vi "HEAT3.vi"() -> ()   [LabVIEW 2020]
uses:
  Control 2.ctl
  TDS_ProccesConfig.ctl
  rga_lv_85/SRSRGA85.llb/SRSRGAo RefNum.ctl
  <vilib>/Utility/miscctls.llb/LVRowAndColumnTypeDef.ctl
  <vilib>/Utility/sysdir.llb/System Directory Type.ctl
  <vilib>/Modbus/master/Create Master Instance (TCP).vi
  <vilib>/Utility/config.llb/Read Key (String).vi
  <vilib>/Waveform/WDTFileIO.llb/Export Waveforms To Spreadsheet File (1D).vi
  <vilib>/Utility/config.llb/Write Key (String).vi
  <vilib>/Modbus/master/Modbus Master.lvclass
  <vilib>/Utility/config.llb/NI_LVConfig.lvlib
panel:
  in  "TDS 2":T1={"Target Temp:"=10.0, "Target Ramp:"=1.0, "Ramp unit:"=1, "Temp. unit:"=0, "Target Ue [V]:"=500.0, "Target Ic [A]:"=2.0, "Heating Mode:"=FALSE, "PID Output:"=FALSE, "Regulation Type"=FALSE, "RGA Specifications"=[{"Mass"=2, "Noise Floor"=4, "CEM "=FALSE}], "Heating Recipe"=[]} {"RGA Specifications"."Noise Floor" min=0 max=7; "RGA Specifications"."Mass" min=1 max=300; "Temp. unit:" items=["K"=1, "C"=0]; "Ramp unit:" items=["/s", "/m", "/h"]}
  in  "TDS":T1={"Target Temp:"=10.0, "Target Ramp:"=1.0, "Ramp unit:"=1, "Temp. unit:"=0, "Target Ue [V]:"=500.0, "Target Ic [A]:"=2.0, "Heating Mode:"=FALSE, "PID Output:"=FALSE, "Regulation Type"=FALSE, "RGA Specifications"=[{"Mass"=2, "Noise Floor"=4, "CEM "=FALSE}], "Heating Recipe"=[]} {"RGA Specifications"."Noise Floor" min=0 max=7; "RGA Specifications"."Mass" min=1 max=300; "Temp. unit:" items=["K"=1, "C"=0]; "Ramp unit:" items=["/s", "/m", "/h"]}
  out "Remote:":bool
  out "heat_LastData":dbl[](array[numeric])
  out "size(s) 3":i32
  out "HEAT start time":timestamp=timestamp(3621395400.2120705 s since 1904-01-01)
  out "Array 2":waveform(dbl)[](array[waveform])
  out "Boolean":T2=TRUE
  out "stopped_loops":bool=TRUE
  in  "Tab Control":T3(tab)
  in  "Start 1":bool=TRUE
  in  "Clear ALL":bool
  out "Waveform Graph":waveform(dbl)[](graph)
  out "main Graph":T4(graph)={"heat_LastData[0]"=21.230000000000018, "heat_LastData[1]"=-273.15, "heat_LastData[2]"=0.0, "heat_LastData[3]"=0.0, "heat_LastData[4]"=0.0, "heat_LastData[5]"=0.0, "heat_LastData[6]"=0.0, "heat_LastData[7]"=0.0, "heat_LastData[8]"=0.0}
  in  "Clear ALL 2":bool
  in  "Start 2":bool=TRUE
  out "main Graph 2":T5(graph)
  in  "Tab Control 2":T6(tab)
  out "DualDC":bool
  out "Text Ring 5":u16(ring) items=["C/s", "C/m", "C/h"]
  out "Act. Ramp:":dbl=1.0
  in  "Save As Button":bool
  in  "Regulation TYpe":bool caption="Regulation Type:"
  in  "Target Ue [V]:":dbl=500.0
  in  "Target Ic [A]:":dbl=2.0
  in  "PID Output:":bool caption="PID Output Signal:"
  in  "Heating Mode:":bool
  out "Text Ring 3":u16(ring) items=["C/s", "C/m", "C/h"]
  out "Interlock:":bool
  out "Operate:":bool
  out "Text Ring":u16(ring) items=["K"=1, "C"=0]
  in  "OperateButton":bool caption="Operate:"
  out "Act. Temp:":dbl=24.100000000000023
  out "Act. P":dbl=100.0
  out "Act. I":dbl=50.0
  out "Act. D":dbl=1.0
  in  "Target Temp:":dbl=10.0
  in  "Target Ramp:":dbl=1.0
  in  "Temp. unit:":u16(ring) items=["K"=1, "C"=0]
  out "Act. Setpoint:":dbl=21.55000000000001
  out "Text Ring 2":u16(ring) items=["K"=1, "C"=0]
  in  "Ramp unit:":u16(ring)=1 items=["/s", "/m", "/h"]
  out "RES active:":bool
  out "EB active:":bool
  in  "Channel:":u16(ring)=7 items=["D1"=9, "D2"=11, "RTD"=13, "TC1"=5, "TC2"=7]
  in  "clean":bool
  out "Operate status::":bool[](array[boolean])=[FALSE, FALSE, FALSE, FALSE, FALSE, TRUE, TRUE, TRUE, FALSE, FALSE, FALSE, TRUE, FALSE, FALSE, FALSE, FALSE]
  in  "Shutter: CH1":bool caption="Shutter:"
  in  "ShutterControl":bool
  in  "Loadproject":bool
  in  "Saveproject":bool
  in  "Sampling time":dbl=250.0 format="%#_g ms"
  in  "Adv.RampControl":bool=TRUE
  out "Connected:":bool=TRUE
  in  "Reconect":bool
  out "Comunication error:":bool
  out "Text Ring 4":u16(ring) items=["C/s", "C/m", "C/h"]
  out "loop time":u32=499
  in  "Lock Button":bool
  in  "address":string="192.168.201.50"
  out "error out":errorcluster
  in  "Default Ramp:":dbl=60.0
  out "ResetActRamp":bool
  out "Uc Act.:":dbl
  out "Ic Act.:":dbl
  out "Uc Act.:":dbl
  out "Ic Act.:":dbl
  out "Ue Act.:":dbl
  out "Ie Act.:":dbl
  in  "Ie limit [mA]:":dbl
  in  "Ue limit [V]:":dbl
  in  "Ic limit [A]:":dbl
  in  "Uc limit [V]:":dbl
  in  "Ic limit:1":dbl caption="Ic limit [A]:"
  in  "Uc limit:1":dbl caption="Uc limit [V]:"
  out "new D":dbl=1.0
  out "new I":dbl=50.0
  out "new P":dbl=100.0
  in  "PID auto tab":string[][](table)
  in  "PID manual setting":string[][](table)=[["100", "50", "1"]]
  in  "Auto PID control":bool=TRUE
  out "New PID request":bool
  in  "Tab Control Duble Res":enum32{"HEAT3 Control", "HEAT3 Limits", "PID"}(tab)
  out "Text Ring 6":u16(ring) items=["K"=1, "C"=0]
  out "Act. Setpoint: 2":dbl=21.55000000000001 caption="Act. Setpoint:"
  in  "Target Ramp: 2":dbl=1.0 caption="Target Ramp:"
  in  "Target Temp: 2":dbl=10.0 caption="Target Temp:"
  out "Act. D 2":dbl=1.0 caption="Act. D"
  out "Act. I 2":dbl=50.0 caption="Act. I"
  out "Act. P 2":dbl=100.0 caption="Act. P"
  out "Act. Temp:":dbl=24.100000000000023
  out "Text Ring 7":u16(ring) items=["K"=1, "C"=0]
  out "Text Ring 8":u16(ring) items=["C/s", "C/m", "C/h"]
  in  "Target Ic [A]: 2":dbl=2.0 caption="Target Ic [A]:"
  out "Act. Ramp: 2":dbl=1.0 caption="Act. Ramp:"
  out "Text Ring 9":u16(ring) items=["C/s", "C/m", "C/h"]
  out "Text Ring 10":u16(ring) items=["K"=1, "C"=0]
  in  "OperateButton 2":bool caption="Operate:"
  in  "Regulation TYpe 2":bool caption="Regulation Type:"
  out "Operate: 2":bool caption="Operate:"
  out "Interlock: 2":bool caption="Interlock:"
  in  "Shutter: CH2":bool caption="Shutter:"
  in  "Uc limit:1 2":dbl caption="Uc limit [V]:"
  in  "Ic limit:1 2":dbl caption="Ic limit [A]:"
  out "Ic Act.: 2":dbl caption="Ic Act.:"
  out "Uc Act.: 2":dbl caption="Uc Act.:"
  out "New PID request 2":bool caption="New PID request"
  in  "Auto PID control 2":bool=TRUE caption="Auto PID control"
  in  "PID manual setting 2":string[][](table)=[["100", "50", "1"]] caption="PID manual setting"
  in  "PID auto tab 2":string[][](table) caption="PID auto tab"
  out "new P 2":dbl=100.0 caption="new P"
  out "new I 2":dbl=50.0 caption="new I"
  out "new D 2":dbl=1.0 caption="new D"
  in  "stop":bool=TRUE
  # "EB:"
  # "Process config.:"
  # "RES:"
  # "EB:"
  # "RES:"
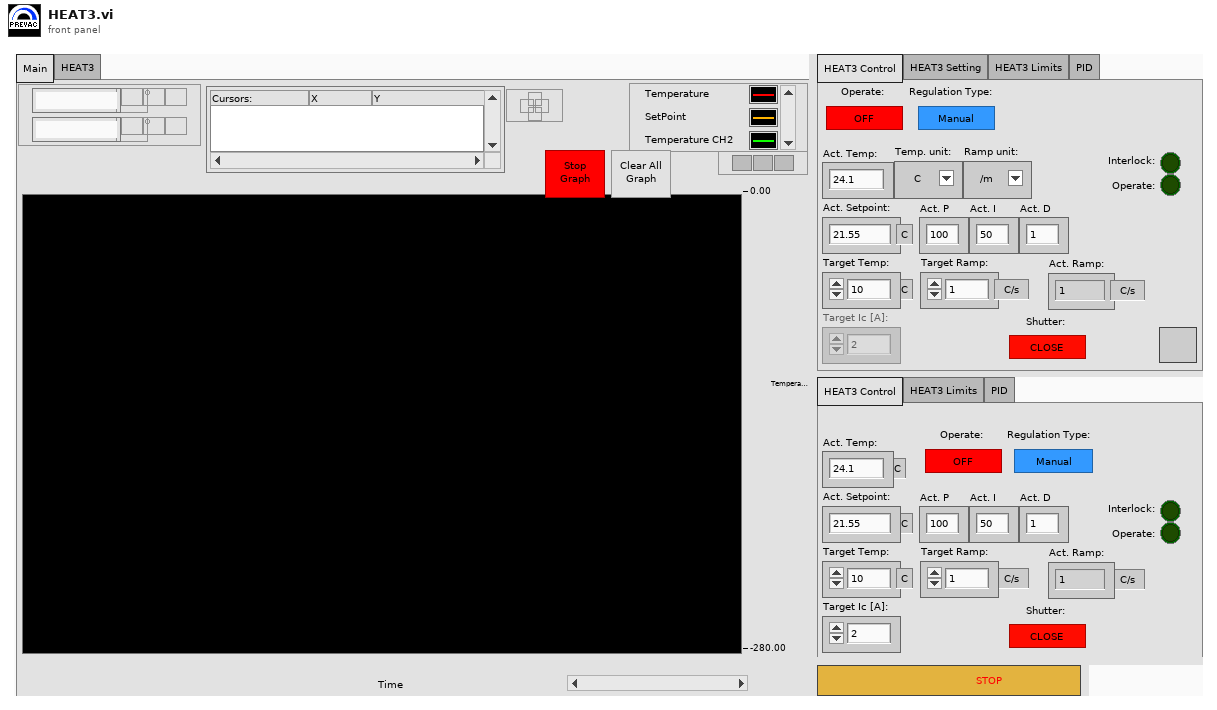
[diagram p1: front panel]
types:
  T1 = typedef "TDS_ProccesConfig.ctl" = cluster{"Target Temp:":dbl, "Target Ramp:":dbl, "Ramp unit:":u16, "Temp. unit:":u16, "Target Ue [V]:":dbl, "Target Ic [A]:":dbl, "Heating Mode:":bool, "PID Output:":bool, "Regulation Type":bool, "RGA Specifications":cluster{"Mass":i32, "Noise Floor":i32, "CEM ":bool}[], "Heating Recipe":cluster{"X":dbl, "Y":dbl}[]}
  T2 = typedef "Control 2.ctl" = bool
  T3 = enum32{"Main", "XY Graph", "Heating recepice", "RGA", "HEAT3"}
  T4 = cluster{"heat_LastData[0]":dbl, "heat_LastData[1]":dbl, "heat_LastData[2]":dbl, "heat_LastData[3]":dbl, "heat_LastData[4]":dbl, "heat_LastData[5]":dbl, "heat_LastData[6]":dbl, "heat_LastData[7]":dbl, "heat_LastData[8]":dbl}
  T5 = cluster{"[0]":dbl, "[1]":dbl, "[2]":dbl, "[3]":dbl}
  T6 = enum32{"HEAT3 Control", "HEAT3 Setting", "HEAT3 Limits", "PID"}
  T7 = typedef "SRSRGAo RefNum.ctl" = u16
  T8 = typedef "LVRowAndColumnTypeDef.ctl" = cluster{"Row":i32, "Column":i32}
  T9 = enum8{"Enabled", "Disabled", "Disabled and Grayed Out"}
  T10 = cluster{"Name":string, "Color":u32, "Style":u8, "Point Style":u8, "Name Visible":bool, "Allow Drag":bool, "Cursor Mode":u32, "Plot":i32, "Index":i32, "Position":cluster{"X":dbl, "Y":dbl}, "X Scale":u32, "Y Scale":u32, "Watch Plots":i32[], "Watch All Plots":bool, "Plot Area":i32, "Label Offset":cluster{"X":dbl, "Y":dbl}}
  T11 = cluster{"heat_LastData[0]":dbl, "heat_LastData[1]":dbl, "heat_LastData[2]":dbl, "heat_LastData[3]":dbl, "heat_LastData[4]":dbl, "heat_LastData[5]":dbl, "heat_LastData[6]":dbl, "heat_LastData[7]":dbl, "heat_LastData[8]":dbl}[]
  T12 = enum16{"open", "replace", "create", "open or create", "replace or create", "replace or create with confirmation"}
  T13 = cluster{"[0]":dbl, "[1]":dbl, "[2]":dbl, "[3]":dbl}[]
  T14 = typedef "LVRectTypeDef.ctl" = cluster{"Left":i16, "Top":i16, "Right":i16, "Bottom":i16}
  T15 = typedef "NI_LVConfig.lvlib/Config Data RefNum.ctl" = refnum<k1>
  T16 = typedef "System Directory Type.ctl" = i32
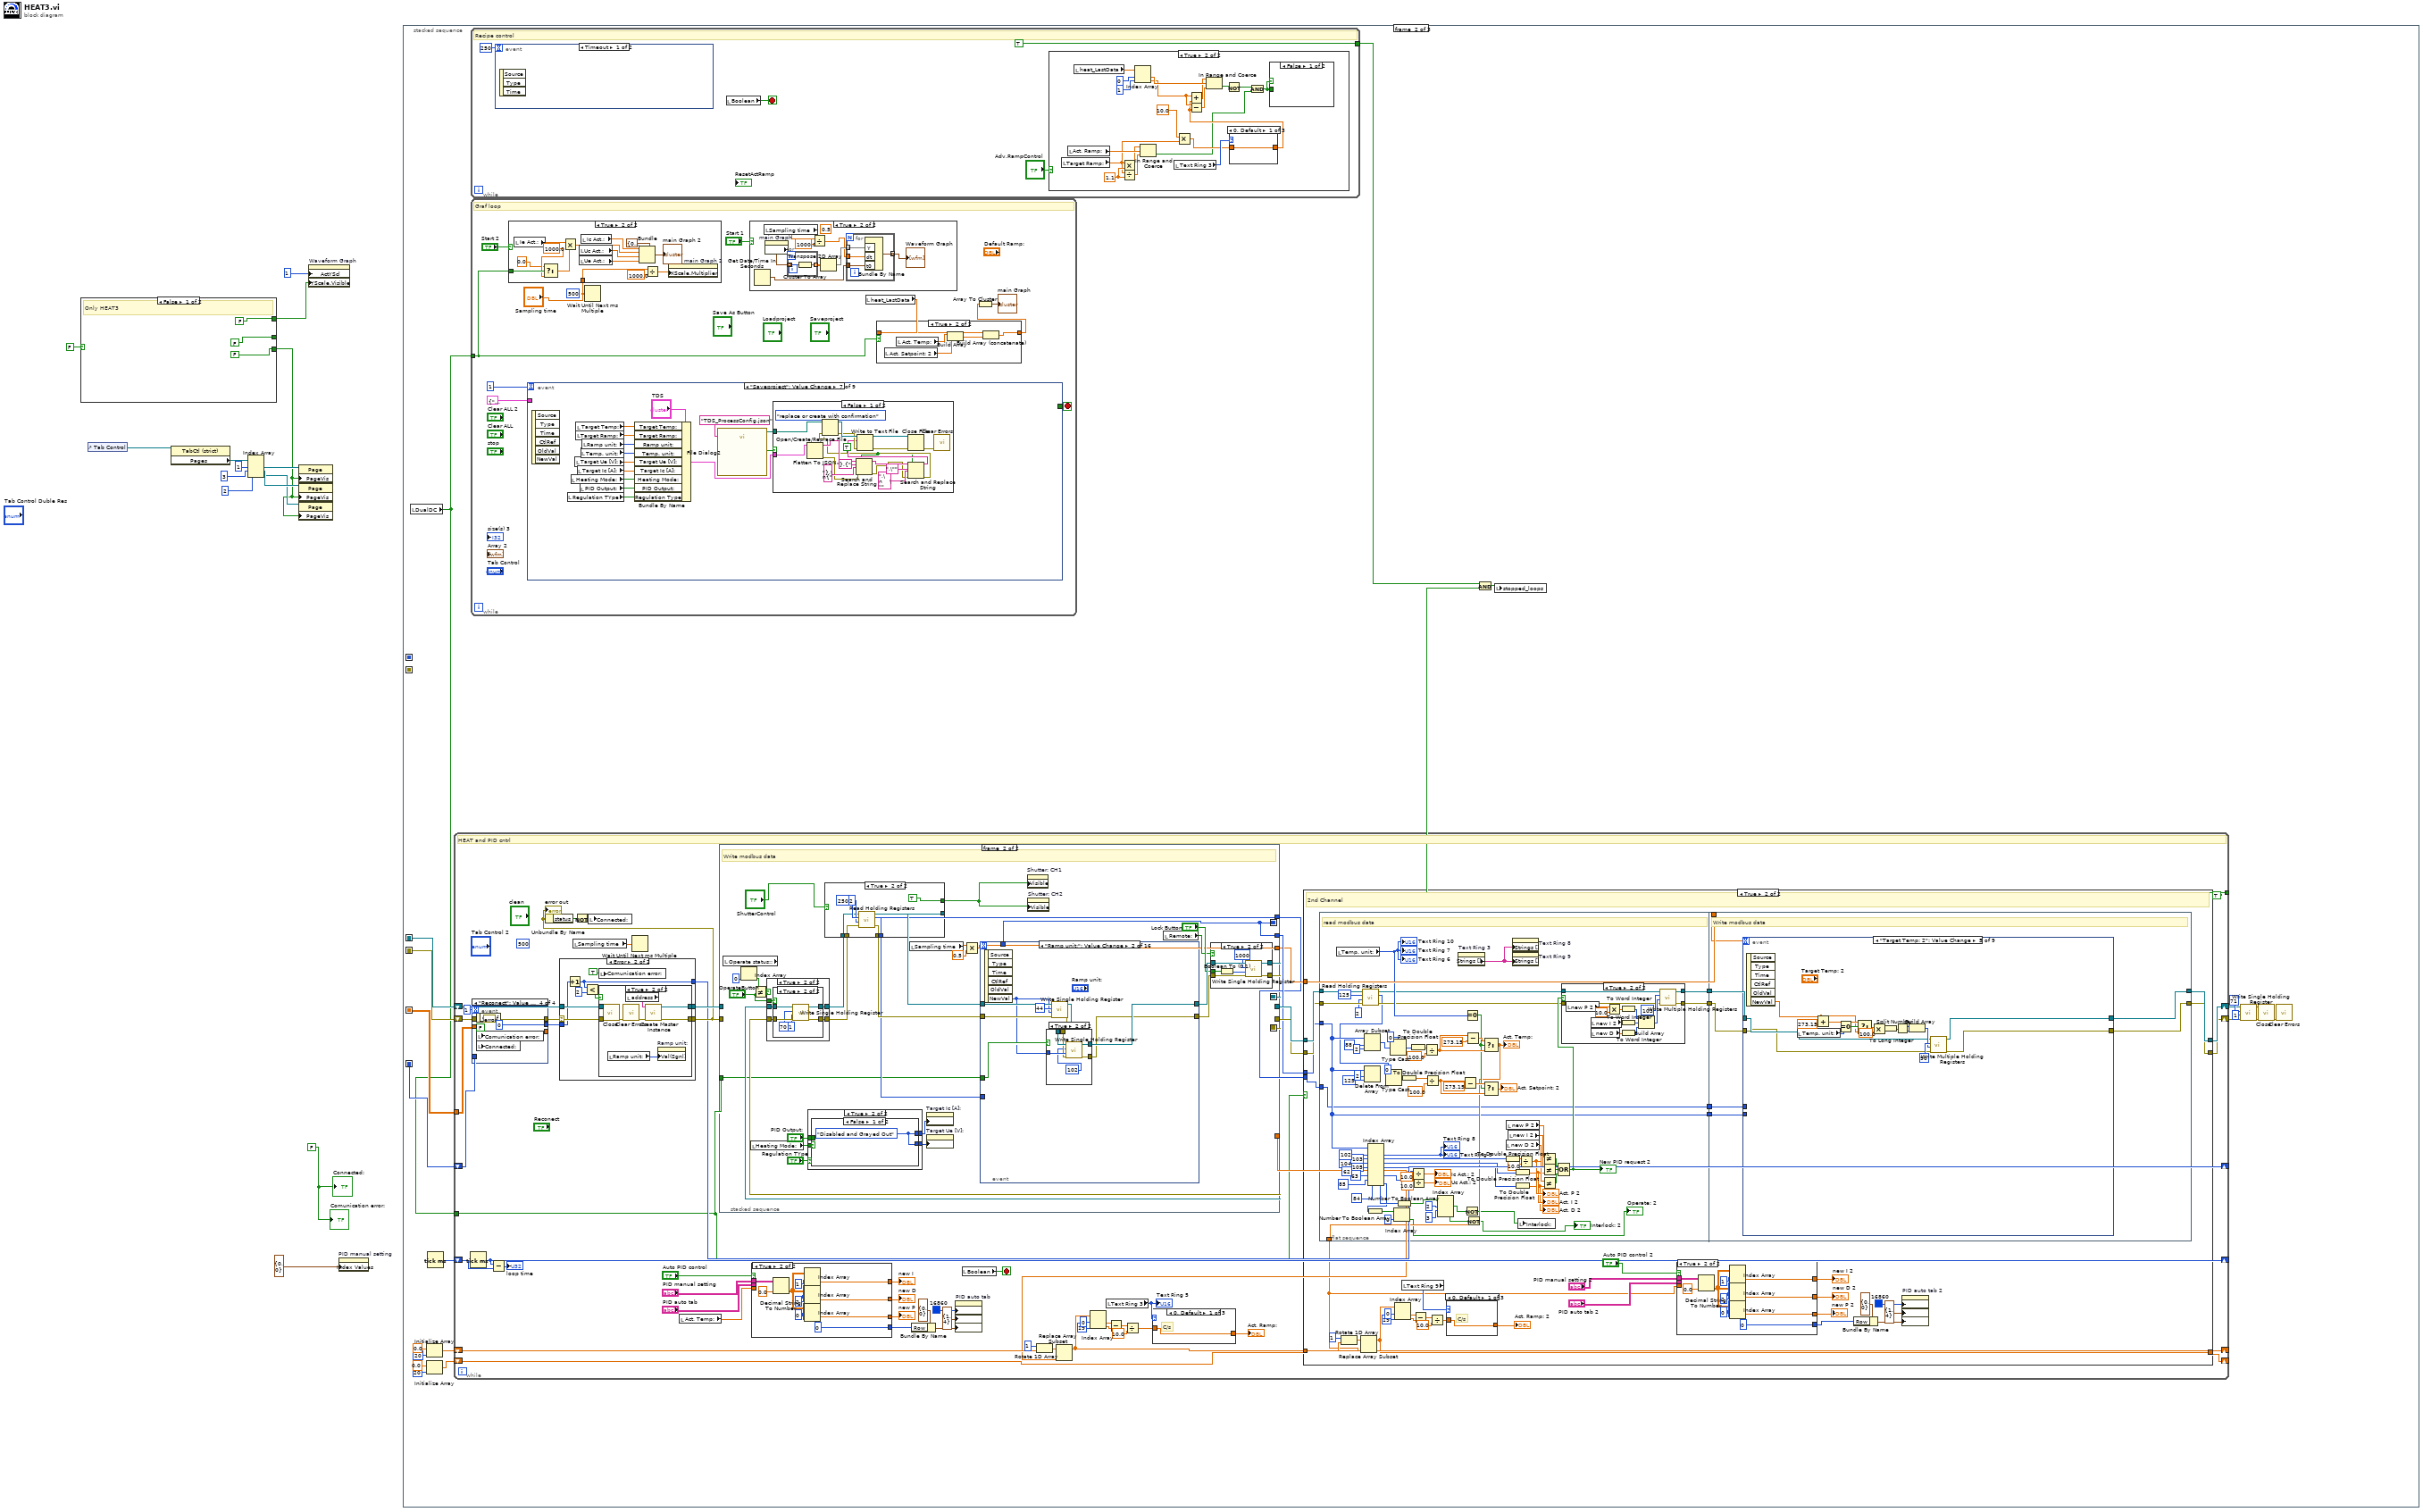
[diagram p0: block diagram]
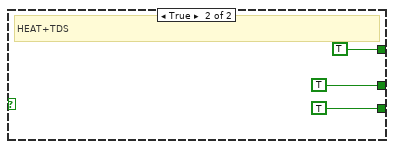
[diagram p2: hidden frame]
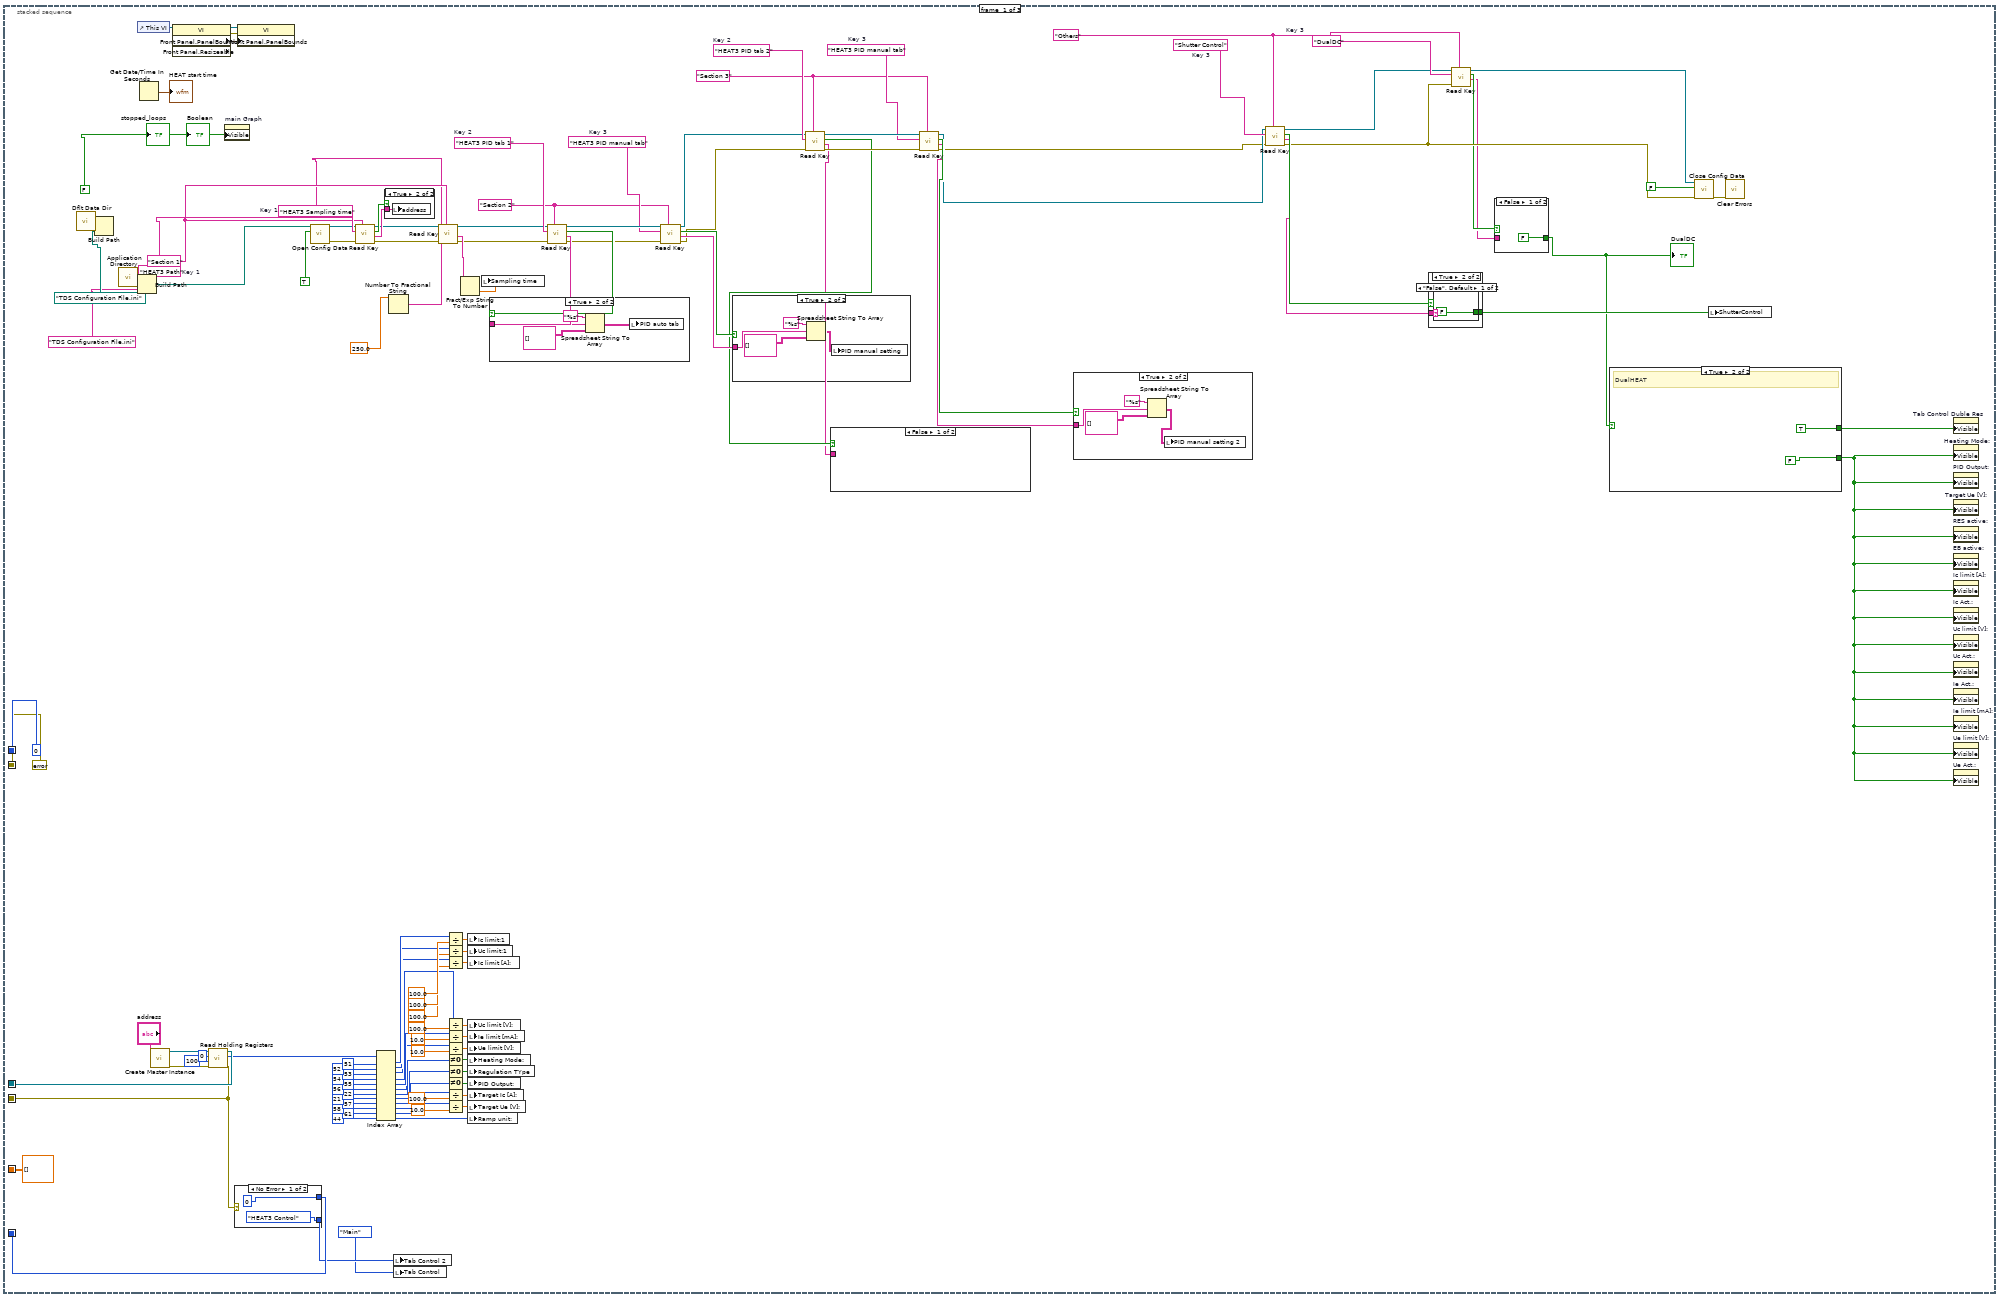
[diagram p3: hidden frame]
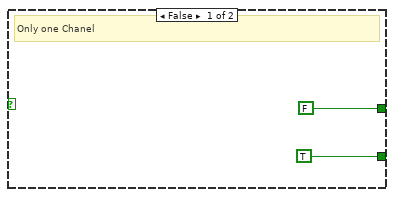
[diagram p4: hidden frame]
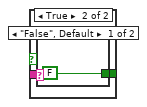
[diagram p5: hidden frame]
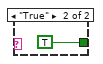
[diagram p6: hidden frame]
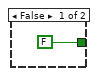
[diagram p7: hidden frame]
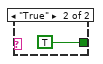
[diagram p8: hidden frame]
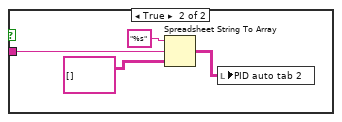
[diagram p10: hidden frame]
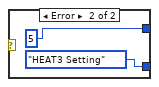
[diagram p13: hidden frame]
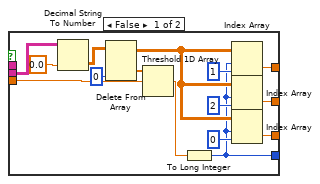
[diagram p16: hidden frame]
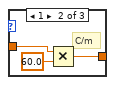
[diagram p17: hidden frame]
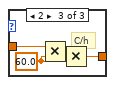
[diagram p18: hidden frame]
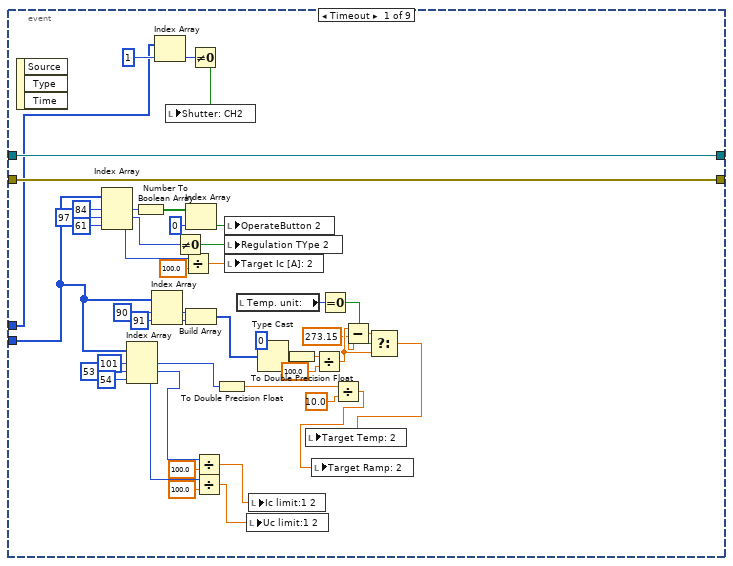
[diagram p20: hidden frame]
diagram:
  w14 = FALSE ("Connected:")
  n1 = case shown="False" FALSE {
    tunnel: [FALSE ("Visible") TRUE ("Visible")] -> _
    tunnel: [FALSE ("Page Visible") TRUE ("Page Visible")] -> w1
    tunnel: [FALSE ("Visible") TRUE ("Visible")] -> w4
    frame False {
      # "Only HEAT3"
    }
    frame True {
      # "HEAT+TDS"
    }
  }
  n2 = control-ref of="Tab Control"() -> (w8:refnum<vi>)
  n3 = property class="TabCtl (strict)"(reference=w8) -> ("Pages"=w11:refnum<vi>[])  [unwired: 1 in, 2 out]
  n4 = Index Array(array=w11, index #1=1 ("index"), index #2=3 ("index"), index #3=2 ("index")) -> (element #1=w9:refnum<vi>, element #2=w6:refnum<vi>, element #3=w2:refnum<vi>)
  n5 = property class="Page"(reference=w9, "PageVis"=w1) -> ()  [unwired: 1 in, 2 out]
  n6 = property class="Page"(reference=w6, "PageVis"=w1) -> ()  [unwired: 1 in, 2 out]
  n7 = property class="Page"(reference=w2, "PageVis"=w1) -> ()  [unwired: 1 in, 2 out]
  n8 = property on="Waveform Graph" class="WFGraph (strict)"("ActYScl"=1, "YScale.Visible"=w4) -> ()  [unwired: 2 in, 2 out]
  n9 = property on="PID manual setting" class="Tbl (strict)"("Index Values"=cluster{"Row":u32, "Column":u32} {"Row"=0, "Column"=0}) -> ()  [unwired: 2 in, 2 out]
  n10 = stacked-sequence {
    seq-local: [w123 _ _] -> [_ w198 _]
    seq-local: [w76 _ _] -> [_ w197 _]
    seq-local: [dbl[][] [] _ _] -> [_ w184 _]
    seq-local: [T7 0 ("SRSRGA Refnum") _ _] -> [_ _ _]
    seq-local: [errorcluster {"status"=FALSE, "code"=0, "source"=""} ("error out") _ _] -> [_ _ _]
    seq-local: [w75 _ _] -> [_ w189 _]
    frame #0 {
      w29 = "DualDC"  # Key 3
      w30 = "Others" ("section")
      w37 = "Shutter Control"  # Key 3
      w44 = "HEAT3 PID manual tab"  # Key 3
      w47 = "HEAT3 PID tab 2"  # Key 2
      w34 = "Section 3" ("section")
      w53 = "HEAT3 Sampling time"  # Key 1
      w68 = "HEAT3 PID manual tab"  # Key 3
      w74 = "HEAT3 PID tab 1"  # Key 2
      w65 = "Section 2" ("section")
      w130 = "HEAT3 Path"  # Key 1
      w54 = "Section 1" ("section")
      w63 = FALSE ("Boolean")
      n11 = call <vilib>:"Dflt Data Dir.vi"() -> ("App:Default Data Directory"=w135:path)
      n12 = Build Path(base path=w135, name or relative path=path "TDS Configuration File.ini" ("default name")) -> ()  [unwired: 1 out]
      n13 = call <vilib>:"Application Directory.vi"() -> ("Application Directory"=w60:path)
      n14 = control-ref of="This VI"() -> (w140:refnum<vi>)
      n15 = Build Path(base path=w60, name or relative path="TDS Configuration File.ini") -> (appended path=w59:path)
      n16 = Get Date/Time In Seconds() -> (seconds since 1Jan1904=→"HEAT start time":timestamp)
      n17 = call-poly <vilib>:"Create Master Instance.vi"("address"="address") -> ("error out"=w124:errorcluster, "TCP master instance"=w125:refnum<class "Modbus Master.lvclass">)  [unwired: 9 in]
      n18 = property class="VI" props=["Front Panel.PanelBounds", "Front Panel.Resizeable"](reference=w140) -> (reference out=w138:refnum<vi>, error out=w137:errorcluster, "Front Panel.PanelBounds"=w139:T14)  [unwired: 1 in, 1 out]
      n19 = call-dynamic "Read Holding Registers.vi"("error in (no error)"=w124, "number of holding registers"=u16 100, "starting address"=u16 0, "Modbus master in"=w125) -> ("error out"=w76:errorcluster, "register values"=w118:u16[], "Modbus master out"=w123:refnum<class "Modbus Master.lvclass">)  [unwired: 5 in]
      n20 = property on="main Graph" class="WFChart (strict)"("Visible"=w63) -> ()  [unwired: 2 in, 2 out]
      n21 = case shown="No Error" w76 {
        tunnel: [0 5] -> w75
        tunnel: [T6."HEAT3 Control" ("Tab Control 2") T6."HEAT3 Setting" ("Tab Control 2")] -> w71
        frame No Error {
        }
        frame Error {
        }
      }
      n22 = property class="VI"(reference=w138, error in=w137, "Front Panel.PanelBounds"=w139) -> ()  [unwired: 2 out]
      n23 = call <vilib>:"Open Config Data.vi"("create file if necessary (T)"=TRUE ("create file if necessary? (T)"), "configuration file path"=w59) -> ("error out"=w128:errorcluster, "refnum"=w129:T15)  [unwired: 7 in, 1 out]
      n24 = call-poly <vilib>:"Read Key.vi"("section"=w54, "error in (no error)"=w128, "key"=w130, "refnum"=w129) -> ("error out"=w50:errorcluster, "value"=w132:string, "found?"=w131:bool, "refnum out"=w52:T15)  [unwired: 2 in, 2 out]
      n25 = Index Array(array=w118, index #1=51 ("index"), index #2=52 ("index"), index #3=53 ("index"), index #4=54 ("index"), index #5=55 ("index"), index #6=56 ("index"), index #7=22 ("index"), index #8=21 ("index"), index #9=57 ("index"), index #10=58 ("index"), index #11=61 ("index"), index #12=44 ("index")) -> (element #1=w109:u16, element #2=w108:u16, element #3=w107:u16, element #4=w95:u16, element #5=w106:u16, element #6=w94:u16, element #7=w98:u16, element #8=w48:u16, element #9=w87:u16, element #10=w80:u16, element #11=w79:u16, element #12=w77:u16)
      n26 = case shown="True" w131 {
        tunnel: w132 -> [_ w177]
        frame False {
        }
        frame True {
          n27 = local write "address"(w177) -> ()
        }
      }
      n28 = Number To Fractional String(number=250.0) -> (F-format string=w57:string)  [unwired: 3 in]
      n29 = local write "Tab Control 2"(w71) -> ()
      n30 = local write "Tab Control"(T3."Main" ("Tab Control")) -> ()
      n31 = call-poly <vilib>:"Read Key.vi"("section"=w54, "error in (no error)"=w50, "default value"=w57, "key"=w53, "refnum"=w52) -> ("error out"=w49:errorcluster, "value"=w56:string, "refnum out"=w51:T15)  [unwired: 1 in, 3 out]
      n32 = Divide(x=w109, y=100.0) -> (x/y=w105:dbl)
      n33 = Divide(x=w108, y=100.0) -> (x/y=w104:dbl)
      n34 = Divide(x=w107, y=100.0) -> (x/y=w103:dbl)
      n35 = Divide(x=w95, y=100.0) -> (x/y=w102:dbl)
      n36 = Divide(x=w106, y=10.0) -> (x/y=w101:dbl)
      n37 = Divide(x=w94, y=10.0) -> (x/y=w100:dbl)
      n38 = Not Equal To 0?(x=w98) -> (x != 0?=w97:bool)
      n39 = Not Equal To 0?(x=w48) -> (x != 0?=w91:bool)
      n40 = Not Equal To 0?(x=w87) -> (x != 0?=w90:bool)
      n41 = Divide(x=w80, y=100.0) -> (x/y=w84:dbl)
      n42 = Divide(x=w79, y=10.0) -> (x/y=w83:dbl)
      n43 = Fract/Exp String To Number(string=w56) -> (number=w55:dbl)  [unwired: 3 in, 1 out]
      n44 = local write "Ic limit:1"(w105) -> ()
      n45 = local write "Uc limit:1"(w104) -> ()
      n46 = local write "Ic limit [A]:"(w103) -> ()
      n47 = local write "Uc limit [V]:"(w102) -> ()
      n48 = local write "Ie limit [mA]:"(w101) -> ()
      n49 = local write "Ue limit [V]:"(w100) -> ()
      n50 = local write "Heating Mode:"(w97) -> ()
      n51 = local write "Regulation TYpe"(w91) -> ()
      n52 = local write "PID Output:"(w90) -> ()
      n53 = local write "Target Ic [A]:"(w84) -> ()
      n54 = local write "Target Ue [V]:"(w83) -> ()
      n55 = local write "Ramp unit:"(w77) -> ()
      n56 = local write "Sampling time"(w55) -> ()
      n57 = call-poly <vilib>:"Read Key.vi"("section"=w65, "error in (no error)"=w49, "key"=w74, "refnum"=w51) -> ("error out"=w69:errorcluster, "value"=w72:string, "found?"=w73:bool, "refnum out"=w70:T15)  [unwired: 2 in, 2 out]
      n58 = case shown="True" w73 {
        tunnel: w72 -> [_ w172]
        frame False {
        }
        frame True {
          n59 = Spreadsheet String To Array(format string="%s", spreadsheet string=w172, array type (2D Dbl)=string[][] [] ("PID auto tab")) -> (array=w169:string[][])  [unwired: 1 in]
          n60 = local write "PID auto tab"(w169) -> ()
        }
      }
      n61 = call-poly <vilib>:"Read Key.vi"("section"=w65, "error in (no error)"=w69, "key"=w68, "refnum"=w70) -> ("error out"=w42:errorcluster, "value"=w66:string, "found?"=w67:bool, "refnum out"=w43:T15)  [unwired: 2 in, 2 out]
      n62 = case shown="True" w67 {
        tunnel: w66 -> [_ w166]
        frame False {
        }
        frame True {
          n63 = Spreadsheet String To Array(format string="%s", spreadsheet string=w166, array type (2D Dbl)=string[][] [] ("PID auto tab")) -> (array=w165:string[][])  [unwired: 1 in]
          n64 = local write "PID manual setting"(w165) -> ()
        }
      }
      n65 = call-poly <vilib>:"Read Key.vi"("section"=w34, "error in (no error)"=w42, "key"=w47, "refnum"=w43) -> ("error out"=w45:errorcluster, "value"=w40:string, "found?"=w41:bool, "refnum out"=w46:T15)  [unwired: 2 in, 2 out]
      n66 = case shown="False" w41 {
        tunnel: w40 -> [_ w164]
        frame False {
        }
        frame True {
          n67 = Spreadsheet String To Array(format string="%s", spreadsheet string=w164, array type (2D Dbl)=string[][] [] ("PID auto tab")) -> (array=w161:string[][])  [unwired: 1 in]
          n68 = local write "PID auto tab 2"(w161) -> ()
        }
      }
      n69 = call-poly <vilib>:"Read Key.vi"("section"=w34, "error in (no error)"=w45, "key"=w44, "refnum"=w46) -> ("error out"=w35:errorcluster, "value"=w38:string, "found?"=w39:bool, "refnum out"=w36:T15)  [unwired: 2 in, 2 out]
      n70 = case shown="True" w39 {
        tunnel: w38 -> [_ w158]
        frame False {
        }
        frame True {
          n71 = Spreadsheet String To Array(format string="%s", spreadsheet string=w158, array type (2D Dbl)=string[][] [] ("PID auto tab")) -> (array=w157:string[][])  [unwired: 1 in]
          n72 = local write "PID manual setting 2"(w157) -> ()
        }
      }
      n73 = call-poly <vilib>:"Read Key.vi"("section"=w30, "error in (no error)"=w35, "key"=w37, "refnum"=w36) -> ("error out"=w26:errorcluster, "value"=w32:string, "found?"=w33:bool, "refnum out"=w28:T15)  [unwired: 2 in, 2 out]
      n74 = case shown="True" w33 {
        tunnel: w32 -> [_ w154]
        tunnel: [FALSE ("Page Visible") w153] -> w31
        frame False {
        }
        frame True {
          n75 = case shown="\"False\", Default" w154 {
            tunnel: [FALSE ("Page Visible") TRUE ("Page Visible")] -> w153
            frame "False", Default {
            }
            frame "True" {
            }
          }
        }
      }
      n76 = call-poly <vilib>:"Read Key.vi"("section"=w30, "error in (no error)"=w26, "key"=w29, "refnum"=w28) -> ("value"=w24:string, "found?"=w25:bool, "refnum out"=w27:T15)  [unwired: 2 in, 3 out]
      n77 = case shown="False" w25 {
        tunnel: w24 -> [_ w149]
        tunnel: [FALSE ("Page Visible") w148] -> w21
        frame False {
        }
        frame True {
          n78 = case shown="\"False\", Default" w149 {
            tunnel: [FALSE ("Page Visible") TRUE ("Page Visible")] -> w148
            frame "False", Default {
            }
            frame "True" {
            }
          }
        }
      }
      "DualDC" <- w21
      n79 = case shown="True" w21 {
        tunnel: [FALSE ("Page Visible") TRUE ("Page Visible")] -> w23
        tunnel: [TRUE ("Page Visible") FALSE ("Page Visible")] -> w22
        frame False {
          # "Only one Chanel"
        }
        frame True {
          # "DualHEAT"
        }
      }
      n80 = call <vilib>:"Close Config Data.vi"("error in (no error)"=w26, "write file if changed (T)"=FALSE ("write configuration file? (T)"), "refnum"=w27) -> ("error out"=w62:errorcluster)  [unwired: 8 out]
      n81 = local write "ShutterControl"(w31) -> ()
      n82 = call <vilib>:"Clear Errors.vi"("error in (no error)"=w62) -> ()  [unwired: 5 in, 2 out]
      n83 = property on="Tab Control Duble Res" class="TabCtl (strict)"("Visible"=w23) -> ()  [unwired: 2 in, 2 out]
      n84 = property on="Heating Mode:" class="Bool (strict)"("Visible"=w22) -> ()  [unwired: 2 in, 2 out]
      n85 = property on="PID Output:" class="Bool (strict)"("Visible"=w22) -> ()  [unwired: 2 in, 2 out]
      n86 = property on="Target Ue [V]:" class="DigNum (strict)"("Visible"=w22) -> ()  [unwired: 2 in, 2 out]
      n87 = property on="RES active:" class="Bool (strict)"("Visible"=w22) -> ()  [unwired: 2 in, 2 out]
      n88 = property on="EB active:" class="Bool (strict)"("Visible"=w22) -> ()  [unwired: 2 in, 2 out]
      n89 = property on="Ic limit [A]:" class="DigNum (strict)"("Visible"=w22) -> ()  [unwired: 2 in, 2 out]
      n90 = property on="Ic Act.:" class="DigNum (strict)"("Visible"=w22) -> ()  [unwired: 2 in, 2 out]
      n91 = property on="Uc limit [V]:" class="DigNum (strict)"("Visible"=w22) -> ()  [unwired: 2 in, 2 out]
      n92 = property on="Uc Act.:" class="DigNum (strict)"("Visible"=w22) -> ()  [unwired: 2 in, 2 out]
      n93 = property on="Ie Act.:" class="DigNum (strict)"("Visible"=w22) -> ()  [unwired: 2 in, 2 out]
      n94 = property on="Ie limit [mA]:" class="DigNum (strict)"("Visible"=w22) -> ()  [unwired: 2 in, 2 out]
      n95 = property on="Ue limit [V]:" class="DigNum (strict)"("Visible"=w22) -> ()  [unwired: 2 in, 2 out]
      n96 = property on="Ue Act.:" class="DigNum (strict)"("Visible"=w22) -> ()  [unwired: 2 in, 2 out]
      "stopped_loops" <- w63
      "Boolean" <- w63
    }
    frame #1 {
      n97 = local read "DualDC"() -> (w178:bool)
      n98 = Initialize Array(0.0 ("element"), 20 ("dimension size")) -> (w179:dbl[])
      n99 = Initialize Array(0.0 ("element"), 20 ("dimension size")) -> (w186:dbl[])
      n100 = Tick Count (ms)() -> (millisecond timer value=w185:u32)
      n101 = while {
        tunnel: [TRUE] -> w182
        shift-right: [w206] -> w193
        shift-left: w197 -> [w232]
        shift-right: [w208] -> w194
        shift-left: w198 -> [w240]
        shift-right: [w236] -> _
        shift-left: w185 -> [w235]
        shift-right: [w225] -> _
        shift-left: w189 -> [w230]
        tunnel: w184 -> [w237]
        shift-right: [w221] -> _
        shift-left: w186 -> [w224]
        tunnel: w178 -> [w204]
        shift-right: [w202] -> _
        shift-left: w179 -> [w203]
        stop <- w253 stop-if-true
        (unwired) u32 500 ("millisecond multiple")
        # "HEAT and PID cntrl"
        n102 = Tick Count (ms)() -> (millisecond timer value=w236:u32)
        n103 = event shown="[3] \"Reconect\": Value Change" {
          selector: _ -> [_ _ _ _]
          dyn-events: _ -> [_ _ _ _]
          timeout: 1 -> [_ _ _ _]
          tunnel: w237 -> [w971 _ _ _]
          tunnel: [w969 dbl[][] [] _ _] -> _
          tunnel: [w968 w974 errorcluster {"status"=TRUE, "code"=0, "source"="Connect to\nnew IP addres"} ("error constant") errorcluster {"status"=TRUE, "code"=0, "source"="Rconnecting"} ("error constant")] -> w231
          tunnel: w232 -> [w968 w974 _ _]
          tunnel: [w967 w973 0 0] -> w229
          tunnel: w230 -> [w967 w973 _ _]
          event Timeout {
            n104 = event-data() -> ()  [unwired: 1 in, 1 out]
            n105 = Select(t=w971, s=FALSE ("build array of data?"), f=dbl[][] []) -> (s? t:f=w969:dbl[][])
          }
          event "clean": Value Change {
            n106 = event-data() -> ()  [unwired: 1 in, 1 out]
            n107 = Get Date/Time In Seconds() -> (seconds since 1Jan1904=w975:timestamp)
            n108 = local write "HEAT start time"(w975) -> ()
            n109 = local write "clean"(FALSE ("clc graph")) -> ()
          }
          event "address": Value Change {
            n110 = event-data() -> ()  [unwired: 1 in, 1 out]
          }
          event "Reconect": Value Change {
            w980 = FALSE ("Connected:")
            n111 = event-data() -> ()  [unwired: 1 in, 1 out]
            n112 = local write "Comunication error:"(w980) -> ()
            n113 = local write "Connected:"(w980) -> ()
          }
        }
        n114 = Subtract(x=w236, y=w235) -> (x-y=→"loop time":u32)
        n115 = case shown="Error" w231 {
          selector: w231 -> [w987 w996]
          tunnel: [w987 w993] -> w227
          tunnel: w240 -> [w986 w995]
          tunnel: [w986 w994] -> w239
          tunnel: w229 -> [_ w991]
          tunnel: [0 w990] -> w225
          frame No Error {
            w983 = FALSE
            n116 = Not(x=w983) -> (.not. x?=w984:bool)
            n117 = local write "Comunication error:"(w983) -> ()
            n118 = local write "Connected:"(w984) -> ()
          }
          frame Error {
            n119 = Increment(x=w991) -> (x+1=w990:i32)
            n120 = Less?(x=w990, y=2) -> (x < y?=w989:bool)
            n121 = local write "Comunication error:"(TRUE) -> ()
            n122 = case shown="True" w989 {
              tunnel: w996 -> [w997 w1006]
              tunnel: w995 -> [w998 w1005]
              tunnel: [w998 w1003] -> w994
              tunnel: [w997 w1002] -> w993
              frame False {
              }
              frame True {
                n123 = call-dynamic "Close.vi"("error in (no error)"=w1006, "Modbus master in"=w1005) -> ("error out"=w1001:errorcluster)  [unwired: 9 in]
                n124 = local read "Ramp unit:"() -> (w999:u16)
                n125 = call <vilib>:"Clear Errors.vi"("error in (no error)"=w1001) -> ("error out"=w1000:errorcluster)  [unwired: 5 in, 1 out]
                n126 = local read "address"() -> (w1004:string)
                n127 = call-poly <vilib>:"Create Master Instance.vi"("error in (no error)"=w1000, "address"=w1004) -> ("error out"=w1002:errorcluster, "TCP master instance"=w1003:refnum<class "Modbus Master.lvclass">)  [unwired: 8 in]
                n128 = property on="Ramp unit:" class="Ring (strict)"("Val(Sgnl)"=w999) -> ()  [unwired: 2 in, 2 out]
              }
            }
          }
        }
        "error out" <- w227
        n129 = Unbundle By Name(w227) -> ("status"=w228:bool)
        n130 = local read "Sampling time"() -> (w211:dbl)
        n131 = Not(x=w228) -> (.not. x?=w226:bool)
        n132 = local write "Connected:"(w226) -> ()
        n133 = Wait Until Next ms Multiple(millisecond multiple=w211) -> ()  [unwired: 1 out]
        n134 = local read "Act. Temp:"() -> (w241:dbl)
        n135 = stacked-sequence {
          seq-local: [w589 _] -> [_ w677]
          seq-local: [w588 _] -> [_ w676]
          seq-local: [w573 _] -> [_ w662]
          tunnel: w239 -> [w587 _]
          tunnel: w227 -> [w586 _]
          tunnel: [_ w669] -> w209
          tunnel: [_ w667] -> w207
          tunnel: [w577 _] -> w210
          tunnel: [_ w662] -> w205
          tunnel: w204 -> [w572 w653]
          tunnel: [_ w661] -> w201
          tunnel: [_ w656] -> w200
          frame #0 {
            # "read modbus data"
            n136 = call-dynamic "Read Holding Registers.vi"("error in (no error)"=w586, "number of holding registers"=u16 1, "starting address"=u16 1151, "Modbus master in"=w587) -> ("error out"=w584:errorcluster, "register values"=w578:u16[], "Modbus master out"=w585:refnum<class "Modbus Master.lvclass">)  [unwired: 5 in]
            n137 = Index Array(array=w578) -> (element=w579:u16)  [unwired: 1 in]
            n138 = Not Equal To 0?(x=w579) -> (x != 0?=w580:bool)
            "Remote:" <- w580
            n139 = case shown="False" w580 {
              tunnel: [T9."Disabled and Grayed Out" ("Disabled") T9."Enabled" ("Disabled")] -> w581
              frame False {
                n140 = local write "Lock Button"(FALSE ("Lock Button")) -> ()
              }
              frame True {
              }
            }
            n141 = local read "Act. Setpoint:"() -> (w605:dbl)
            n142 = disable-structure shown="Disabled" {
              disable-tunnel: [w634 u16 2] -> w610
              frame Disabled {
                n143 = Decrement(x="Channel:") -> (x-1=w634:u16)
              }
              frame Enabled {
              }
            }
            n144 = local read "Act. Temp:"() -> (w577:dbl)
            n145 = call-dynamic "Read Holding Registers.vi"("error in (no error)"=w584, "number of holding registers"=u16 1, "starting address"=u16 0, "Modbus master in"=w585) -> ("error out"=w622:errorcluster, "register values"=w594:u16[], "Modbus master out"=w623:refnum<class "Modbus Master.lvclass">)  [unwired: 5 in]
            n146 = property on="Lock Button" class="Bool (strict)"("DisabledEnum"=w581) -> ()  [unwired: 2 in, 2 out]
            n147 = call-dynamic "Read Holding Registers.vi"("error in (no error)"=w622, "number of holding registers"=u16 2, "starting address"=w610, "Modbus master in"=w623) -> ("error out"=w628:errorcluster, "register values"=w608:u16[], "Modbus master out"=w629:refnum<class "Modbus Master.lvclass">)  [unwired: 5 in]
            n148 = call "Modbus_Get_Status_list.vi"("register values"=w594) -> ("Boolean"=w602:bool, "Boolean 2"=→"Operate:":bool, "Boolean array"=→"Operate status::":bool[])  [unwired: 8 in]
            n149 = Build Array(w577, w605) -> (→"heat_LastData":dbl[])
            n150 = Not(x=w602) -> (.not. x?=→"Interlock:":bool)
            n151 = local read "new D"() -> (w618:dbl)
            n152 = local read "new P"() -> (w616:dbl)
            n153 = local read "new I"() -> (w620:dbl)
            n154 = call-dynamic "Read Holding Registers.vi"("error in (no error)"=w628, "number of holding registers"=u16 3, "starting address"=u16 45, "Modbus master in"=w629) -> ("error out"=w612:errorcluster, "register values"=w596:u16[], "Modbus master out"=w614:refnum<class "Modbus Master.lvclass">)  [unwired: 5 in]
            n155 = Select(t=u16 125 ("number of holding registers"), s=w572, f=u16 125 ("number of holding registers")) -> (s? t:f=w569:u16)
            n156 = call "Modbus_Pid_Control.vi"("register values"=w596, "new D"=w618, "new I"=w620, "new P"=w616) -> ("Numeric"=→"Act. D":dbl, "Numeric 2"=→"Act. I":dbl, "Numeric 3"=→"Act. P":dbl, "Boolean"=w595:bool)  [unwired: 4 in]
            "New PID request" <- w595
            n157 = call-dynamic "Read Holding Registers.vi"("error in (no error)"=w612, "number of holding registers"=w569, "starting address"=u16 0, "Modbus master in"=w614) -> ("error out"=w611:errorcluster, "register values"=w573:u16[], "Modbus master out"=w613:refnum<class "Modbus Master.lvclass">)  [unwired: 5 in]
            n158 = local read "Temp. unit:"() -> (w607:u16)
            n159 = case shown="True" w595 {
              tunnel: w613 -> [w637 w642]
              tunnel: w611 -> [w638 w641]
              tunnel: [w637 w640] -> w589
              tunnel: [w638 w639] -> w588
              frame False {
              }
              frame True {
                n160 = local read "new P"() -> (w650:dbl)
                n161 = local read "new D"() -> (w652:dbl)
                n162 = local read "new I"() -> (w651:dbl)
                n163 = Multiply(x=w650, y=10.0) -> (x*y=w646:dbl)
                n164 = To Word Integer(number=w646) -> (16bit integer=w647:i16)
                n165 = To Word Integer(number=w651) -> (16bit integer=w648:i16)
                n166 = To Word Integer(number=w652) -> (16bit integer=w649:i16)
                n167 = Build Array(w647, w648, w649) -> (w643:i16[])
                n168 = call-dynamic "Write Multiple Holding Registers.vi"("error in (no error)"=w641, "holding register values"=w643, "starting address"=u16 45, "Modbus master in"=w642) -> ("error out"=w639:errorcluster, "Modbus master out"=w640:refnum<class "Modbus Master.lvclass">)  [unwired: 6 in]
              }
            }
            n169 = Index Array(array=w573, index=22) -> (element=w592:u16)
            n170 = call "Modbus_Get_Temp.vi"("register values"=w608, "Temp. unit:"="Temp. unit:") -> ("Numeric"=→"Act. Temp:":dbl, "Strings []"=w574:string[])  [unwired: 8 in]
            n171 = Not Equal To 0?(x=w592) -> (x != 0?=w591:bool)
            "EB active:" <- w591
            n172 = property on="Text Ring 3" class="Ring (strict)"("Strings []"=w574) -> ()  [unwired: 2 in, 2 out]
            n173 = call "Modbus_Decode_Multiple_registers.vi"("Temp. unit:"=w607, "register values"=w573) -> ("Numeric 3"=→"Uc Act.:" →"Uc Act.:":dbl, "Numeric 4"=→"Ic Act.:" →"Ic Act.:":dbl, "Numeric 5"=→"Act. Setpoint:":dbl, "Numeric 2"=→"Ie Act.:":dbl, "register"=→"Text Ring 3" →"Text Ring 4":u16, "Numeric"=→"Ue Act.:":dbl)  [unwired: 4 in]
            n174 = Not(x=w591) -> (.not. x?=→"RES active:":bool)
            n175 = property on="Text Ring 5" class="Ring (strict)"("Strings []"=w574) -> ()  [unwired: 2 in, 2 out]
            "Text Ring" <- "Temp. unit:"
            "Text Ring 2" <- "Temp. unit:"
          }
          frame #1 {
            # "Write modbus data"
            n176 = local read "Operate status::"() -> (w682:bool[])
            n177 = Index Array(array=w682, index=0) -> (element=w680:bool)
            n178 = local read "Heating Mode:"() -> (w672:bool)
            n179 = Not Equal?(x=w680, y="OperateButton") -> (x != y?=w679:bool)
            n180 = case shown="True" w679 {
              tunnel: w677 -> [w949 w954]
              tunnel: w676 -> [w948 w953]
              tunnel: [w949 w952] -> w660
              tunnel: [w948 w951] -> w659
              tunnel: "OperateButton" -> [_ w950]
              frame False {
              }
              frame True {
                n181 = case shown="True" w950 {
                  tunnel: w954 -> [w958 w966]
                  tunnel: w953 -> [w957 w965]
                  tunnel: [w956 w964] -> w952
                  tunnel: [w955 w963] -> w951
                  frame False {
                    n182 = call-dynamic "Write Single Holding Register.vi"("error in (no error)"=w957, "holding register value"=u16 1, "address"=u16 71, "Modbus master in"=w958) -> ("error out"=w955:errorcluster, "Modbus master out"=w956:refnum<class "Modbus Master.lvclass">)  [unwired: 6 in]
                  }
                  frame True {
                    n183 = call-dynamic "Write Single Holding Register.vi"("error in (no error)"=w965, "holding register value"=u16 1, "address"=u16 70, "Modbus master in"=w966) -> ("error out"=w963:errorcluster, "Modbus master out"=w964:refnum<class "Modbus Master.lvclass">)  [unwired: 6 in]
                  }
                }
              }
            }
            n184 = case shown="True" "Regulation TYpe" {
              tunnel: [w705 w713] -> w674
              tunnel: [w704 w712] -> w673
              tunnel: w672 -> [w706 w711]
              tunnel: "PID Output:" -> [_ w710]
              frame False {
                n185 = case shown="True" w706 {
                  tunnel: [T9."Enabled" ("Disabled") w709] -> w705
                  tunnel: [T9."Disabled and Grayed Out" ("Disabled") w709] -> w704
                  frame False {
                  }
                  frame True {
                    w709 = T9."Enabled" ("Disabled")
                  }
                }
              }
              frame True {
                n186 = case shown="False" w711 {
                  tunnel: [w714 w716] -> w713
                  tunnel: [w714 w715] -> w712
                  tunnel: w710 -> [_ w717]
                  frame False {
                    w714 = T9."Disabled and Grayed Out" ("Disabled")
                  }
                  frame True {
                    n187 = case shown="False" w717 {
                      tunnel: [T9."Enabled" ("Disabled") T9."Disabled and Grayed Out" ("Disabled")] -> w716
                      tunnel: [T9."Disabled and Grayed Out" ("Disabled") T9."Enabled" ("Disabled")] -> w715
                      frame False {
                      }
                      frame True {
                      }
                    }
                  }
                }
              }
            }
            n188 = case shown="True" "ShutterControl" {
              tunnel: w660 -> [w685 w692]
              tunnel: w659 -> [w686 w691]
              tunnel: [w686 w690] -> w658
              tunnel: [w685 w689] -> w657
              tunnel: [i32[] [0, 0] w688] -> w656
              tunnel: [FALSE TRUE] -> w655
              frame False {
              }
              frame True {
                n189 = call-dynamic "Read Holding Registers.vi"("error in (no error)"=w691, "number of holding registers"=u16 2, "starting address"=u16 250, "Modbus master in"=w692) -> ("error out"=w690:errorcluster, "register values"=w688:u16[], "Modbus master out"=w689:refnum<class "Modbus Master.lvclass">)  [unwired: 5 in]
              }
            }
            n190 = local read "Sampling time"() -> (w664:dbl)
            n191 = property on="Target Ic [A]:" class="DigNum (strict)"("DisabledEnum"=w674) -> ()  [unwired: 2 in, 2 out]
            n192 = property on="Target Ue [V]:" class="DigNum (strict)"("DisabledEnum"=w673) -> ()  [unwired: 2 in, 2 out]
            n193 = Multiply(x=w664, y=0.5) -> (x*y=w661:dbl)
            n194 = event shown="[1] \"Ramp unit:\": Value Change" {
              selector: _ -> [_ _ _ _ _ _ _ _ _ _ _ _ _ _ _ _]
              dyn-events: _ -> [_ _ _ _ _ _ _ _ _ _ _ _ _ _ _ _]
              timeout: w661 -> [_ _ _ _ _ _ _ _ _ _ _ _ _ _ _ _]
              tunnel: w657 -> [w727 w807 w822 w831 w840 w849 w858 w867 w876 w885 w893 w901 w909 w928 w936 w943]
              tunnel: [w725 w800 w823 w832 w841 w850 w859 w868 w877 w886 w894 w902 w910 w925 w937 w940] -> w668
              tunnel: w658 -> [w724 w806 w821 w830 w839 w848 w857 w866 w875 w884 w892 w900 w908 w927 w935 w942]
              tunnel: [w726 w801 w824 w833 w842 w851 w860 w869 w878 w887 w895 w903 w911 w926 w938 w941] -> w670
              tunnel: w662 -> [w723 _ _ _ _ _ _ _ _ _ _ _ _ _ _ _]
              tunnel: w656 -> [w722 _ _ _ _ _ _ _ _ _ _ _ _ _ _ _]
              tunnel: w653 -> [_ w805 _ _ _ _ _ _ _ _ _ _ _ _ _ _]
              event Timeout {
                n195 = event-data() -> ()  [unwired: 1 in, 3 out]
                n196 = case shown="No Error" w724 {
                  tunnel: w727 -> [w733 w799]
                  tunnel: w724 -> [w732 w798]
                  tunnel: [w733 w799] -> w726
                  tunnel: [w732 w798] -> w725
                  tunnel: w723 -> [w734 _]
                  tunnel: w722 -> [w730 _]
                  frame No Error {
                    n197 = Index Array(array=w734, index #1=51 ("index"), index #2=52 ("index"), index #3=53 ("index"), index #4=54 ("index"), index #5=55 ("index"), index #6=56 ("index"), index #7=u16 44 ("address")) -> (element #1=w776:u16, element #2=w777:u16, element #3=w778:u16, element #4=w780:u16, element #5=w779:u16, element #6=w756:u16, element #7=w755:u16)
                    n198 = Index Array(array=w734, index #1=u16 22 ("address"), index #2=u16 57 ("address"), index #3=u16 21 ("address"), index #4=u16 58 ("address"), index #5=61 ("index")) -> (element #1=w796:u16, element #2=w793:u16, element #3=w790:u16, element #4=w787:u16, element #5=w783:u16)
                    n199 = Index Array(array=w730, index=u16 0 ("address")) -> (element=w729:i32)
                    n200 = Index Array(array=w734, index=u16 43 ("address")) -> (element=w737:u16)
                    n201 = Not Equal To 0?(x=w790) -> (x != 0?=w791:bool)
                    n202 = Index Array(array=w734, index #1=u16 14 ("address"), index #2=u16 15 ("address")) -> (element #1=w752:u16, element #2=w751:u16)
                    n203 = Not Equal To 0?(x=w796) -> (x != 0?=w797:bool)
                    n204 = Not Equal To 0?(x=w729) -> (x != 0?=w728:bool)
                    n205 = Divide(x=w783, y=10.0) -> (x/y=w785:dbl)
                    n206 = Divide(x=w787, y=100.0) -> (x/y=w788:dbl)
                    n207 = Divide(x=w776, y=100.0) -> (x/y=w758:dbl)
                    n208 = Divide(x=w777, y=100.0) -> (x/y=w759:dbl)
                    n209 = Divide(x=w778, y=100.0) -> (x/y=w760:dbl)
                    n210 = Divide(x=w780, y=100.0) -> (x/y=w761:dbl)
                    n211 = Divide(x=w779, y=10.0) -> (x/y=w762:dbl)
                    n212 = Divide(x=w756, y=10.0) -> (x/y=w763:dbl)
                    n213 = Not Equal To 0?(x=w793) -> (x != 0?=w794:bool)
                    n214 = local write "Regulation TYpe"(w791) -> ()
                    n215 = Build Array(w752, w751) -> (w740:u16[])
                    n216 = local write "Heating Mode:"(w797) -> ()
                    n217 = local write "Target Ue [V]:"(w785) -> ()
                    n218 = local write "Shutter: CH1"(w728) -> ()
                    n219 = local write "Target Ic [A]:"(w788) -> ()
                    n220 = local write "PID Output:"(w794) -> ()
                    n221 = local write "Ic limit [A]:"(w760) -> ()
                    n222 = local write "Ic limit:1"(w758) -> ()
                    n223 = local write "Uc limit:1"(w759) -> ()
                    n224 = local write "Uc limit [V]:"(w761) -> ()
                    n225 = local write "Ie limit [mA]:"(w762) -> ()
                    n226 = local write "Ue limit [V]:"(w763) -> ()
                    n227 = local write "Ramp unit:"(w755) -> ()
                    n228 = To Double Precision Float(number=w737) -> (double precision float=w736:dbl)
                    n229 = local read "Temp. unit:"() -> (w749:u16)
                    n230 = Type Cast(type=0, x=w740) -> (*(type *) &x=w748:i32)
                    n231 = To Double Precision Float(number=w748) -> (double precision float=w747:dbl)
                    n232 = Divide(x=w747, y=100.0) -> (x/y=w746:dbl)
                    n233 = Equal To 0?(x=w749) -> (x = 0?=w744:bool)
                    n234 = Divide(x=w736, y=10.0) -> (x/y=w735:dbl)
                    n235 = Subtract(x=w746, y=273.15) -> (x-y=w745:dbl)
                    n236 = local write "Target Ramp:"(w735) -> ()
                    n237 = Select(t=w745, s=w744, f=w746) -> (s? t:f=w750:dbl)
                    n238 = local write "Target Temp:"(w750) -> ()
                  }
                  frame Error {
                  }
                }
              }
              event "Ramp unit:": Value Change {
                n239 = event-data() -> ("NewVal"=w804:u16)  [unwired: 1 in, 5 out]
                n240 = call-dynamic "Write Single Holding Register.vi"("error in (no error)"=w806, "holding register value"=w804, "address"=u16 44, "Modbus master in"=w807) -> ("error out"=w803:errorcluster, "Modbus master out"=w802:refnum<class "Modbus Master.lvclass">)  [unwired: 6 in]
                n241 = case shown="True" w805 {
                  tunnel: w804 -> [_ w816]
                  tunnel: w802 -> [w810 w815]
                  tunnel: w803 -> [w809 w814]
                  tunnel: [w810 w813] -> w801
                  tunnel: [w809 w812] -> w800
                  frame False {
                  }
                  frame True {
                    n242 = call-dynamic "Write Single Holding Register.vi"("error in (no error)"=w814, "holding register value"=w816, "address"=u16 102, "Modbus master in"=w815) -> ("error out"=w812:errorcluster, "Modbus master out"=w813:refnum<class "Modbus Master.lvclass">)  [unwired: 6 in]
                  }
                }
              }
              event "Ic limit:1": Value Change {
                n243 = event-data() -> ("NewVal"=w818:dbl)  [unwired: 1 in, 5 out]
                n244 = Multiply(x=w818, y=100.0) -> (x*y=w820:dbl)
                n245 = To Unsigned Word Integer(number=w820) -> (unsigned 16bit integer=w817:u16)
                n246 = call-dynamic "Write Single Holding Register.vi"("error in (no error)"=w821, "holding register value"=w817, "address"=u16 51, "Modbus master in"=w822) -> ("error out"=w823:errorcluster, "Modbus master out"=w824:refnum<class "Modbus Master.lvclass">)  [unwired: 6 in]
              }
              event "Uc limit:1": Value Change {
                n247 = event-data() -> ("NewVal"=w827:dbl)  [unwired: 1 in, 5 out]
                n248 = Multiply(x=w827, y=100.0) -> (x*y=w829:dbl)
                n249 = To Unsigned Word Integer(number=w829) -> (unsigned 16bit integer=w826:u16)
                n250 = call-dynamic "Write Single Holding Register.vi"("error in (no error)"=w830, "holding register value"=w826, "address"=u16 52, "Modbus master in"=w831) -> ("error out"=w832:errorcluster, "Modbus master out"=w833:refnum<class "Modbus Master.lvclass">)  [unwired: 6 in]
              }
              event "Ic limit [A]:": Value Change {
                n251 = event-data() -> ("NewVal"=w836:dbl)  [unwired: 1 in, 5 out]
                n252 = Multiply(x=w836, y=100.0) -> (x*y=w838:dbl)
                n253 = To Unsigned Word Integer(number=w838) -> (unsigned 16bit integer=w835:u16)
                n254 = call-dynamic "Write Single Holding Register.vi"("error in (no error)"=w839, "holding register value"=w835, "address"=u16 53, "Modbus master in"=w840) -> ("error out"=w841:errorcluster, "Modbus master out"=w842:refnum<class "Modbus Master.lvclass">)  [unwired: 6 in]
              }
              event "Uc limit [V]:": Value Change {
                n255 = event-data() -> ("NewVal"=w845:dbl)  [unwired: 1 in, 5 out]
                n256 = Multiply(x=w845, y=100.0) -> (x*y=w847:dbl)
                n257 = To Unsigned Word Integer(number=w847) -> (unsigned 16bit integer=w844:u16)
                n258 = call-dynamic "Write Single Holding Register.vi"("error in (no error)"=w848, "holding register value"=w844, "address"=u16 54, "Modbus master in"=w849) -> ("error out"=w850:errorcluster, "Modbus master out"=w851:refnum<class "Modbus Master.lvclass">)  [unwired: 6 in]
              }
              event "Ie limit [mA]:": Value Change {
                n259 = event-data() -> ("NewVal"=w854:dbl)  [unwired: 1 in, 5 out]
                n260 = Multiply(x=w854, y=10.0) -> (x*y=w856:dbl)
                n261 = To Unsigned Word Integer(number=w856) -> (unsigned 16bit integer=w853:u16)
                n262 = call-dynamic "Write Single Holding Register.vi"("error in (no error)"=w857, "holding register value"=w853, "address"=u16 55, "Modbus master in"=w858) -> ("error out"=w859:errorcluster, "Modbus master out"=w860:refnum<class "Modbus Master.lvclass">)  [unwired: 6 in]
              }
              event "Ue limit [V]:": Value Change {
                n263 = event-data() -> ("NewVal"=w863:dbl)  [unwired: 1 in, 5 out]
                n264 = Multiply(x=w863, y=10.0) -> (x*y=w865:dbl)
                n265 = To Unsigned Word Integer(number=w865) -> (unsigned 16bit integer=w862:u16)
                n266 = call-dynamic "Write Single Holding Register.vi"("error in (no error)"=w866, "holding register value"=w862, "address"=u16 56, "Modbus master in"=w867) -> ("error out"=w868:errorcluster, "Modbus master out"=w869:refnum<class "Modbus Master.lvclass">)  [unwired: 6 in]
              }
              event "Target Ue [V]:": Value Change {
                n267 = event-data() -> ("NewVal"=w872:dbl)  [unwired: 1 in, 5 out]
                n268 = Multiply(x=w872, y=10.0) -> (x*y=w874:dbl)
                n269 = To Unsigned Word Integer(number=w874) -> (unsigned 16bit integer=w871:u16)
                n270 = call-dynamic "Write Single Holding Register.vi"("error in (no error)"=w875, "holding register value"=w871, "address"=u16 61, "Modbus master in"=w876) -> ("error out"=w877:errorcluster, "Modbus master out"=w878:refnum<class "Modbus Master.lvclass">)  [unwired: 6 in]
              }
              event "Target Ic [A]:": Value Change {
                n271 = event-data() -> ("NewVal"=w881:dbl)  [unwired: 1 in, 5 out]
                n272 = Multiply(x=w881, y=100.0) -> (x*y=w883:dbl)
                n273 = To Unsigned Word Integer(number=w883) -> (unsigned 16bit integer=w880:u16)
                n274 = call-dynamic "Write Single Holding Register.vi"("error in (no error)"=w884, "holding register value"=w880, "address"=u16 58, "Modbus master in"=w885) -> ("error out"=w886:errorcluster, "Modbus master out"=w887:refnum<class "Modbus Master.lvclass">)  [unwired: 6 in]
              }
              event "Heating Mode:": Value Change {
                n275 = event-data() -> ("NewVal"=w890:bool)  [unwired: 1 in, 5 out]
                n276 = Boolean To (0,1)(Boolean=w890) -> (0, 1=w889:i16)
                n277 = To Unsigned Word Integer(number=w889) -> (unsigned 16bit integer=w891:u16)
                n278 = call-dynamic "Write Single Holding Register.vi"("error in (no error)"=w892, "holding register value"=w891, "address"=u16 22, "Modbus master in"=w893) -> ("error out"=w894:errorcluster, "Modbus master out"=w895:refnum<class "Modbus Master.lvclass">)  [unwired: 6 in]
              }
              event "Regulation TYpe": Value Change {
                n279 = event-data() -> ("NewVal"=w898:bool)  [unwired: 1 in, 5 out]
                n280 = Boolean To (0,1)(Boolean=w898) -> (0, 1=w897:i16)
                n281 = To Unsigned Word Integer(number=w897) -> (unsigned 16bit integer=w899:u16)
                n282 = call-dynamic "Write Single Holding Register.vi"("error in (no error)"=w900, "holding register value"=w899, "address"=u16 21, "Modbus master in"=w901) -> ("error out"=w902:errorcluster, "Modbus master out"=w903:refnum<class "Modbus Master.lvclass">)  [unwired: 6 in]
              }
              event "PID Output:": Value Change {
                n283 = event-data() -> ("NewVal"=w906:bool)  [unwired: 1 in, 5 out]
                n284 = Boolean To (0,1)(Boolean=w906) -> (0, 1=w905:i16)
                n285 = To Unsigned Word Integer(number=w905) -> (unsigned 16bit integer=w907:u16)
                n286 = call-dynamic "Write Single Holding Register.vi"("error in (no error)"=w908, "holding register value"=w907, "address"=u16 57, "Modbus master in"=w909) -> ("error out"=w910:errorcluster, "Modbus master out"=w911:refnum<class "Modbus Master.lvclass">)  [unwired: 6 in]
              }
              event "Target Temp:": Value Change {
                n287 = event-data() -> ("NewVal"=w929:dbl)  [unwired: 1 in, 5 out]
                n288 = local read "Temp. unit:"() -> (w913:u16)
                n289 = Add(x=w929, y=273.15) -> (x+y=w915:dbl)
                n290 = Equal To 0?(x=w913) -> (x = 0?=w916:bool)
                n291 = Select(t=w915, s=w916, f=w929) -> (s? t:f=w914:dbl)
                n292 = Multiply(x=w914, y=100.0) -> (x*y=w923:dbl)
                n293 = To Long Integer(number=w923) -> (32bit integer=w922:i32)
                n294 = Split Number(x=w922) -> (hi(x)=w921:u16, lo(x)=w920:u16)
                n295 = Build Array(w921, w920) -> (w918:u16[])
                n296 = call-dynamic "Write Multiple Holding Registers.vi"("error in (no error)"=w927, "holding register values"=w918, "starting address"=u16 14 ("address"), "Modbus master in"=w928) -> ("error out"=w925:errorcluster, "Modbus master out"=w926:refnum<class "Modbus Master.lvclass">)  [unwired: 6 in]
              }
              event "Target Ramp:": Value Change {
                n297 = event-data() -> ("NewVal"=w939:dbl)  [unwired: 1 in, 5 out]
                n298 = Multiply(x=w939, y=10.0) -> (x*y=w932:dbl)
                n299 = To Word Integer(number=w932) -> (16bit integer=w931:i16)
                n300 = Build Array(w931) -> (w930:i16[])
                n301 = call-dynamic "Write Multiple Holding Registers.vi"("error in (no error)"=w935, "holding register values"=w930, "starting address"=u16 43 ("address"), "Modbus master in"=w936) -> ("error out"=w937:errorcluster, "Modbus master out"=w938:refnum<class "Modbus Master.lvclass">)  [unwired: 6 in]
              }
              event "Shutter: CH1": Value Change {
                n302 = event-data() -> ("NewVal"=w944:bool)  [unwired: 1 in, 5 out]
                n303 = Boolean To (0,1)(Boolean=w944) -> (0, 1=w945:i16)
                n304 = To Unsigned Word Integer(number=w945) -> (unsigned 16bit integer=w946:u16)
                n305 = call-dynamic "Write Single Holding Register.vi"("error in (no error)"=w942, "holding register value"=w946, "address"=u16 250, "Modbus master in"=w943) -> ("error out"=w940:errorcluster, "Modbus master out"=w941:refnum<class "Modbus Master.lvclass">)  [unwired: 6 in]
              }
            }
            n306 = property on="Shutter: CH1" class="Bool (strict)"("Visible"=w655) -> ()  [unwired: 2 in, 2 out]
            n307 = property on="Shutter: CH2" class="Bool (strict)"("Visible"=w655) -> ()  [unwired: 2 in, 2 out]
            n308 = local read "Remote:"() -> (w665:bool)
            n309 = case shown="True" w665 {
              tunnel: w670 -> [w696 w703]
              tunnel: [w696 w702] -> w669
              tunnel: "Lock Button" -> [_ w700]
              tunnel: w668 -> [w695 w698]
              tunnel: [w695 w697] -> w667
              frame False {
              }
              frame True {
                n310 = Boolean To (0,1)(Boolean=w700) -> (0, 1=w699:i16)
                n311 = call-dynamic "Write Single Holding Register.vi"("error in (no error)"=w698, "holding register value"=w699, "address"=1000 ("index"), "Modbus master in"=w703) -> ("error out"=w697:errorcluster, "Modbus master out"=w702:refnum<class "Modbus Master.lvclass">)  [unwired: 6 in]
              }
            }
          }
        }
        n312 = case shown="True" "Auto PID control" {
          tunnel: "PID manual setting" -> [_ w1031]
          tunnel: "PID auto tab" -> [w1020 _]
          tunnel: [w1011 w1026] -> w249
          tunnel: [w1010 w1025] -> w248
          tunnel: [w1009 w1024] -> w247
          tunnel: w241 -> [w1013 _]
          tunnel: [w1007 0] -> w242
          frame False {
            n313 = Decimal String To Number(string=w1020, default (0L)=0.0) -> (number=w1015:dbl[][])  [unwired: 1 in, 1 out]
            n314 = Delete From Array(array=w1015, index (col)=0 ("disabled index (col)")) -> (deleted portion=w1012:dbl[], array with subset deleted=w1014:dbl[][])  [unwired: 2 in]
            n315 = Threshold 1D Array(2:w1013, 3:w1012) -> (0:w1008:dbl)  [unwired: 1 in]
            n316 = To Long Integer(number=w1008) -> (32bit integer=w1007:i32)
            n317 = Index Array(array=w1014, index (row)=w1007, index (col)=1 ("disabled index (col)")) -> (element=w1010:dbl)
            n318 = Index Array(array=w1014, index (row)=w1007, index (col)=2 ("disabled index (col)")) -> (element=w1009:dbl)
            n319 = Index Array(array=w1014, index (row)=w1007, index (col)=0 ("disabled index (col)")) -> (element=w1011:dbl)
          }
          frame True {
            w1027 = 0 ("disabled index (col)")
            n320 = Decimal String To Number(string=w1031, default (0L)=0.0) -> (number=w1023:dbl[][])  [unwired: 1 in, 1 out]
            n321 = Index Array(array=w1023, index (row)=w1027, index (col)=1 ("disabled index (col)")) -> (element=w1025:dbl)
            n322 = Index Array(array=w1023, index (row)=w1027, index (col)=2 ("disabled index (col)")) -> (element=w1024:dbl)
            n323 = Index Array(array=w1023, index (row)=w1027, index (col)=w1027) -> (element=w1026:dbl)
          }
        }
        "new P" <- w249
        "new I" <- w248
        "new D" <- w247
        n324 = Bundle By Name(cluster=T8 {"Row"=0, "Column"=0} ("Selection Start"), "Row"=w242) -> (w243:T8)
        n325 = property on="PID auto tab" class="Tbl (strict)"("Selection Color"=u32 16860, "Selection Size"=T8 {"Row"=1, "Column"=4}, "Selection Start"=w243) -> ()  [unwired: 2 in, 2 out]
        n326 = local read "Boolean"() -> (w253:T2)
        n327 = Rotate 1D Array(1:w224, 2:1 ("n")) -> (0:w222:dbl[])
        n328 = Replace Array Subset(array=w222, new element=w210) -> (w221:dbl[])  [unwired: 1 in]
        n329 = Index Array(array=w221, index #1=0 ("n"), index #2=19 ("n")) -> (element #1=w217:dbl, element #2=w218:dbl)
        n330 = local read "Text Ring 3"() -> (w213:u16)
        "Text Ring 5" <- w213
        n331 = Subtract(x=w217, y=w218) -> (x-y=w216:dbl)
        n332 = Divide(x=w216, y=10.0) -> (x/y=w214:dbl)
        n333 = case shown="0, Default" w213 {
          tunnel: w214 -> [w560 w563 w567]
          tunnel: [w560 w561 w564] -> w212
          frame 0, Default {
            # "C/s"
          }
          frame 1 {
            # "C/m"
            n334 = Multiply(x=w563, y=60.0) -> (x*y=w561:dbl)
          }
          frame 2 {
            w565 = 60.0 ("y")
            # "C/h"
            n335 = Multiply(x=w567, y=w565) -> (x*y=w566:dbl)
            n336 = Multiply(x=w566, y=w565) -> (x*y=w564:dbl)
          }
        }
        "Act. Ramp:" <- w212
        n337 = case shown="True" w204 {
          tunnel: w209 -> [w256 w292]
          tunnel: w207 -> [w255 w291]
          tunnel: [w256 w290] -> w208
          tunnel: [w255 w289] -> w206
          tunnel: w205 -> [_ w288]
          tunnel: w203 -> [w254 w262]
          tunnel: [w254 w275] -> w202
          tunnel: w201 -> [_ w260]
          tunnel: w200 -> [_ w258]
          frame False {
            # "No duall heat"
          }
          frame True {
            # "2nd Channel"
            n338 = flat-sequence {
              tunnel: w292 -> [w333]
              tunnel: w291 -> [w332]
              tunnel: w288 -> [w348]
              tunnel: [w371] -> w287
              tunnel: [w370] -> w286
              tunnel: [w358] -> w261
              tunnel: [w348] -> w259
              tunnel: w258 -> [w326]
              tunnel: [w326] -> w257
              tunnel: [w424] -> w290
              tunnel: [w425] -> w289
              tunnel: w287 -> [w422]
              tunnel: w286 -> [w421]
              tunnel: w260 -> [w423]
              tunnel: w259 -> [w420]
              tunnel: w257 -> [w419]
              frame #0 {
                # "read modbus data"
                n339 = local read "Temp. unit:"() -> (w389:u16)
                "Text Ring 10" <- w389
                "Text Ring 7" <- w389
                "Text Ring 6" <- w389
                n340 = call-dynamic "Read Holding Registers.vi"("error in (no error)"=w332, "number of holding registers"=2 ("length"), "starting address"=125 ("index"), "Modbus master in"=w333) -> ("error out"=w330:errorcluster, "register values"=w327:u16[], "Modbus master out"=w331:refnum<class "Modbus Master.lvclass">)  [unwired: 5 in]
                n341 = Delete From Array(array=w348, length=2, index=125) -> ()  [unwired: 2 out]
                n342 = Array Subset(array=w348, index=88, length=2) -> (w392:u16[])
                n343 = Index Array(array=w348, index #1=102 ("index"), index #2=103 ("index"), index #3=104 ("index"), index #4=105 ("index"), index #5=62 ("index"), index #6=63 ("index"), index #7=85 ("index"), index #8=84 ("index")) -> (element #1=→"Text Ring 8" →"Text Ring 9":u16, element #2=w374:u16, element #3=w373:u16, element #4=w372:u16, element #5=w353:u16, element #6=w350:u16, element #7=w346:u16, element #8=w336:u16)
                n344 = Number To Boolean Array(number=w336) -> (Boolean array=w337:bool[])
                n345 = Type Cast(type=0, x=w327) -> (*(type *) &x=w362:i32)
                n346 = Type Cast(type=0, x=w392) -> (*(type *) &x=w394:i32)
                n347 = Index Array(array=w337, index=0) -> (element=→"Operate: 2":bool)
                n348 = Number To Boolean Array(number=w346) -> (Boolean array=w343:bool[])
                n349 = To Double Precision Float(number=w362) -> (double precision float=w367:dbl)
                n350 = To Double Precision Float(number=w394) -> (double precision float=w396:dbl)
                n351 = Divide(x=w353, y=10.0) -> (x/y=→"Ic Act.: 2":dbl)
                n352 = Divide(x=w350, y=10.0) -> (x/y=→"Uc Act.: 2":dbl)
                n353 = Divide(x=w396, y=100.0) -> (x/y=w397:dbl)
                n354 = Divide(x=w367, y=100.0) -> (x/y=w364:dbl)
                n355 = Index Array(array=w343, index #1=2 ("index"), index #2=3 ("index")) -> (element #1=w342:bool, element #2=w339:bool)  [unwired: 1 in, 1 out]
                n356 = property on="Text Ring 3" class="Ring (strict)"() -> ("Strings []"=w400:string[])  [unwired: 2 in, 2 out]
                n357 = Subtract(x=w364, y=273.15) -> (x-y=w366:dbl)
                n358 = Not(x=w342) -> (.not. x?=w341:bool)
                n359 = Equal To 0?(x=w389) -> (x = 0?=w360:bool)
                n360 = Subtract(x=w397, y=273.15) -> (x-y=w399:dbl)
                n361 = Not(x=w339) -> (.not. x?=→"Interlock: 2":bool)
                n362 = Select(t=w399, s=w360, f=w397) -> (s? t:f=w358:dbl)
                "Act. Temp:" <- w358
                n363 = Select(t=w366, s=w360, f=w364) -> (s? t:f=→"Act. Setpoint: 2":dbl)
                n364 = To Double Precision Float(number=w374) -> (double precision float=w385:dbl)
                n365 = local read "new D 2"() -> (w381:dbl)
                n366 = local read "new P 2"() -> (w383:dbl)
                n367 = local read "new I 2"() -> (w382:dbl)
                n368 = property on="Text Ring 8" class="Ring (strict)"("Strings []"=w400) -> ()  [unwired: 2 in, 2 out]
                n369 = property on="Text Ring 9" class="Ring (strict)"("Strings []"=w400) -> ()  [unwired: 2 in, 2 out]
                n370 = To Double Precision Float(number=w373) -> (double precision float=w379:dbl)
                "Act. I 2" <- w379
                n371 = To Double Precision Float(number=w372) -> (double precision float=w378:dbl)
                "Act. D 2" <- w378
                n372 = local write "Interlock:"(w341) -> ()
                n373 = Divide(x=w385, y=10.0) -> (x/y=w380:dbl)
                "Act. P 2" <- w380
                n374 = Not Equal?(x=w383, y=w380) -> (x != y?=w386:bool)
                n375 = Not Equal?(x=w382, y=w379) -> (x != y?=w387:bool)
                n376 = Not Equal?(x=w381, y=w378) -> (x != y?=w388:bool)
                n377 = Compound Arithmetic op=OR(w386, w387, w388) -> (w357:bool)
                "New PID request 2" <- w357
                n378 = case shown="True" w357 {
                  tunnel: w331 -> [w403 w408]
                  tunnel: w330 -> [w404 w407]
                  tunnel: [w403 w406] -> w371
                  tunnel: [w404 w405] -> w370
                  frame False {
                  }
                  frame True {
                    n379 = local read "new P 2"() -> (w416:dbl)
                    n380 = local read "new I 2"() -> (w417:dbl)
                    n381 = local read "new D"() -> (w418:dbl)
                    n382 = Multiply(x=w416, y=10.0) -> (x*y=w412:dbl)
                    n383 = To Word Integer(number=w412) -> (16bit integer=w413:i16)
                    n384 = To Word Integer(number=w417) -> (16bit integer=w414:i16)
                    n385 = To Word Integer(number=w418) -> (16bit integer=w415:i16)
                    n386 = Build Array(w413, w414, w415) -> (w409:i16[])
                    n387 = call-dynamic "Write Multiple Holding Registers.vi"("error in (no error)"=w407, "holding register values"=w409, "starting address"=u16 103, "Modbus master in"=w408) -> ("error out"=w405:errorcluster, "Modbus master out"=w406:refnum<class "Modbus Master.lvclass">)  [unwired: 6 in]
                  }
                }
              }
              frame #1 {
                # "Write modbus data"
                n388 = event shown="[4] \"Target Temp: 2\": Value Change" {
                  selector: _ -> [_ _ _ _ _ _ _ _ _]
                  dyn-events: _ -> [_ _ _ _ _ _ _ _ _]
                  timeout: w423 -> [_ _ _ _ _ _ _ _ _]
                  tunnel: w422 -> [w472 w474 w493 w501 w511 w527 w537 w546 w555]
                  tunnel: w421 -> [w471 w473 w492 w500 w510 w526 w536 w545 w554]
                  tunnel: [w472 w476 w491 w499 w509 w525 w535 w544 w553] -> w424
                  tunnel: [w471 w475 w490 w498 w508 w524 w534 w543 w552] -> w425
                  tunnel: w420 -> [w426 _ _ _ _ _ _ _ _]
                  tunnel: w419 -> [w428 _ _ _ _ _ _ _ _]
                  event Timeout {
                    n389 = event-data() -> ()  [unwired: 1 in, 3 out]
                    n390 = Index Array(array=w426, index #1=84 ("index"), index #2=97 ("index"), index #3=61 ("index")) -> (element #1=w469:u16, element #2=w464:u16, element #3=w461:u16)
                    n391 = Index Array(array=w426, index #1=u16 101 ("address"), index #2=u16 53 ("address"), index #3=u16 54 ("address")) -> (element #1=w443:u16, element #2=w434:u16, element #3=w433:u16)
                    n392 = Number To Boolean Array(number=w469) -> (Boolean array=w467:bool[])
                    n393 = Index Array(array=w426, index #1=u16 90 ("address"), index #2=u16 91 ("address")) -> (element #1=w456:u16, element #2=w455:u16)
                    n394 = Index Array(array=w428, index=u16 1 ("address")) -> (element=w429:i32)
                    n395 = Not Equal To 0?(x=w464) -> (x != 0?=w463:bool)
                    n396 = Divide(x=w461, y=100.0) -> (x/y=w460:dbl)
                    n397 = Index Array(array=w467, index=0) -> (element=w466:bool)
                    n398 = Build Array(w456, w455) -> (w446:u16[])
                    n399 = Not Equal To 0?(x=w429) -> (x != 0?=w427:bool)
                    n400 = local write "Shutter: CH2"(w427) -> ()
                    n401 = Divide(x=w434, y=100.0) -> (x/y=w432:dbl)
                    n402 = Divide(x=w433, y=100.0) -> (x/y=w431:dbl)
                    n403 = To Double Precision Float(number=w443) -> (double precision float=w442:dbl)
                    n404 = local write "OperateButton 2"(w466) -> ()
                    n405 = local write "Regulation TYpe 2"(w463) -> ()
                    n406 = local write "Target Ic [A]: 2"(w460) -> ()
                    n407 = local read "Temp. unit:"() -> (w441:u16)
                    n408 = local write "Uc limit:1 2"(w431) -> ()
                    n409 = local write "Ic limit:1 2"(w432) -> ()
                    n410 = Type Cast(type=0, x=w446) -> (*(type *) &x=w454:i32)
                    n411 = To Double Precision Float(number=w454) -> (double precision float=w453:dbl)
                    n412 = Divide(x=w453, y=100.0) -> (x/y=w452:dbl)
                    n413 = Equal To 0?(x=w441) -> (x = 0?=w450:bool)
                    n414 = Divide(x=w442, y=10.0) -> (x/y=w439:dbl)
                    n415 = local write "Target Ramp: 2"(w439) -> ()
                    n416 = Subtract(x=w452, y=273.15) -> (x-y=w451:dbl)
                    n417 = Select(t=w451, s=w450, f=w452) -> (s? t:f=w440:dbl)
                    n418 = local write "Target Temp: 2"(w440) -> ()
                  }
                  event "OperateButton 2": Value Change {
                    n419 = event-data() -> ("NewVal"=w477:bool)  [unwired: 1 in, 5 out]
                    n420 = case shown="False" w477 {
                      tunnel: w474 -> [w481 w488]
                      tunnel: [w479 w486] -> w476
                      tunnel: [w478 w485] -> w475
                      tunnel: w473 -> [w480 w484]
                      frame False {
                        n421 = call-dynamic "Write Single Holding Register.vi"("error in (no error)"=w480, "holding register value"=u16 1, "address"=u16 115, "Modbus master in"=w481) -> ("error out"=w478:errorcluster, "Modbus master out"=w479:refnum<class "Modbus Master.lvclass">)  [unwired: 6 in]
                      }
                      frame True {
                        n422 = call-dynamic "Write Single Holding Register.vi"("error in (no error)"=w484, "holding register value"=u16 1, "address"=u16 114, "Modbus master in"=w488) -> ("error out"=w485:errorcluster, "Modbus master out"=w486:refnum<class "Modbus Master.lvclass">)  [unwired: 6 in]
                      }
                    }
                  }
                  event "Regulation TYpe 2": Value Change {
                    n423 = event-data() -> ("NewVal"=w494:bool)  [unwired: 1 in, 5 out]
                    n424 = Boolean To (0,1)(Boolean=w494) -> (0, 1=w495:i16)
                    n425 = To Unsigned Word Integer(number=w495) -> (unsigned 16bit integer=w496:u16)
                    n426 = call-dynamic "Write Single Holding Register.vi"("error in (no error)"=w492, "holding register value"=w496, "address"=u16 97, "Modbus master in"=w493) -> ("error out"=w490:errorcluster, "Modbus master out"=w491:refnum<class "Modbus Master.lvclass">)  [unwired: 6 in]
                  }
                  event "Target Ic [A]: 2": Value Change {
                    n427 = event-data() -> ("NewVal"=w502:dbl)  [unwired: 1 in, 5 out]
                    n428 = Multiply(x=w502, y=100.0) -> (x*y=w505:dbl)
                    n429 = To Unsigned Word Integer(number=w505) -> (unsigned 16bit integer=w503:u16)
                    n430 = call-dynamic "Write Single Holding Register.vi"("error in (no error)"=w500, "holding register value"=w503, "address"=u16 58, "Modbus master in"=w501) -> ("error out"=w498:errorcluster, "Modbus master out"=w499:refnum<class "Modbus Master.lvclass">)  [unwired: 6 in]
                  }
                  event "Target Temp: 2": Value Change {
                    n431 = event-data() -> ("NewVal"=w512:dbl)  [unwired: 1 in, 5 out]
                    n432 = local read "Temp. unit:"() -> (w507:u16)
                    n433 = Add(x=w512, y=273.15) -> (x+y=w514:dbl)
                    n434 = Equal To 0?(x=w507) -> (x = 0?=w515:bool)
                    n435 = Select(t=w514, s=w515, f=w512) -> (s? t:f=w513:dbl)
                    n436 = Multiply(x=w513, y=100.0) -> (x*y=w522:dbl)
                    n437 = To Long Integer(number=w522) -> (32bit integer=w521:i32)
                    n438 = Split Number(x=w521) -> (hi(x)=w520:u16, lo(x)=w519:u16)
                    n439 = Build Array(w520, w519) -> (w517:u16[])
                    n440 = call-dynamic "Write Multiple Holding Registers.vi"("error in (no error)"=w510, "holding register values"=w517, "starting address"=u16 90 ("address"), "Modbus master in"=w511) -> ("error out"=w508:errorcluster, "Modbus master out"=w509:refnum<class "Modbus Master.lvclass">)  [unwired: 6 in]
                  }
                  event "Target Ramp: 2": Value Change {
                    n441 = event-data() -> ("NewVal"=w528:dbl)  [unwired: 1 in, 5 out]
                    n442 = Multiply(x=w528, y=10.0) -> (x*y=w531:dbl)
                    n443 = To Word Integer(number=w531) -> (16bit integer=w530:i16)
                    n444 = Build Array(w530) -> (w529:i16[])
                    n445 = call-dynamic "Write Multiple Holding Registers.vi"("error in (no error)"=w526, "holding register values"=w529, "starting address"=u16 101 ("address"), "Modbus master in"=w527) -> ("error out"=w524:errorcluster, "Modbus master out"=w525:refnum<class "Modbus Master.lvclass">)  [unwired: 6 in]
                  }
                  event "Ic limit:1 2": Value Change {
                    n446 = event-data() -> ("NewVal"=w538:dbl)  [unwired: 1 in, 5 out]
                    n447 = Multiply(x=w538, y=100.0) -> (x*y=w541:dbl)
                    n448 = To Unsigned Word Integer(number=w541) -> (unsigned 16bit integer=w539:u16)
                    n449 = call-dynamic "Write Single Holding Register.vi"("error in (no error)"=w536, "holding register value"=w539, "address"=u16 53, "Modbus master in"=w537) -> ("error out"=w534:errorcluster, "Modbus master out"=w535:refnum<class "Modbus Master.lvclass">)  [unwired: 6 in]
                  }
                  event "Uc limit:1 2": Value Change {
                    n450 = event-data() -> ("NewVal"=w547:dbl)  [unwired: 1 in, 5 out]
                    n451 = Multiply(x=w547, y=100.0) -> (x*y=w550:dbl)
                    n452 = To Unsigned Word Integer(number=w550) -> (unsigned 16bit integer=w548:u16)
                    n453 = call-dynamic "Write Single Holding Register.vi"("error in (no error)"=w545, "holding register value"=w548, "address"=u16 54, "Modbus master in"=w546) -> ("error out"=w543:errorcluster, "Modbus master out"=w544:refnum<class "Modbus Master.lvclass">)  [unwired: 6 in]
                  }
                  event "Shutter: CH2": Value Change {
                    n454 = event-data() -> ("NewVal"=w556:bool)  [unwired: 1 in, 5 out]
                    n455 = Boolean To (0,1)(Boolean=w556) -> (0, 1=w557:i16)
                    n456 = To Unsigned Word Integer(number=w557) -> (unsigned 16bit integer=w558:u16)
                    n457 = call-dynamic "Write Single Holding Register.vi"("error in (no error)"=w554, "holding register value"=w558, "address"=u16 251, "Modbus master in"=w555) -> ("error out"=w552:errorcluster, "Modbus master out"=w553:refnum<class "Modbus Master.lvclass">)  [unwired: 6 in]
                  }
                }
              }
            }
            n458 = Rotate 1D Array(1:w262, 2:1 ("n")) -> (0:w284:dbl[])
            n459 = Replace Array Subset(array=w284, new element=w261) -> (w275:dbl[])  [unwired: 1 in]
            n460 = Index Array(array=w275, index #1=0 ("n"), index #2=19 ("n")) -> (element #1=w280:dbl, element #2=w281:dbl)
            n461 = local read "Text Ring 9"() -> (w263:u16)
            n462 = Subtract(x=w280, y=w281) -> (x-y=w279:dbl)
            n463 = Divide(x=w279, y=10.0) -> (x/y=w277:dbl)
            n464 = case shown="0, Default" w263 {
              tunnel: w277 -> [w318 w321 w325]
              tunnel: [w318 w319 w322] -> w276
              frame 0, Default {
                # "C/s"
              }
              frame 1 {
                # "C/m"
                n465 = Multiply(x=w321, y=60.0) -> (x*y=w319:dbl)
              }
              frame 2 {
                w323 = 60.0 ("y")
                # "C/h"
                n466 = Multiply(x=w325, y=w323) -> (x*y=w324:dbl)
                n467 = Multiply(x=w324, y=w323) -> (x*y=w322:dbl)
              }
            }
            "Act. Ramp: 2" <- w276
            n468 = case shown="True" "Auto PID control 2" {
              tunnel: "PID manual setting 2" -> [_ w317]
              tunnel: "PID auto tab 2" -> [w306 _]
              tunnel: [w297 w312] -> w269
              tunnel: [w296 w311] -> w268
              tunnel: [w295 w310] -> w267
              tunnel: w261 -> [w299 _]
              tunnel: [w293 0] -> w273
              frame False {
                n469 = Decimal String To Number(string=w306, default (0L)=0.0) -> (number=w301:dbl[][])  [unwired: 1 in, 1 out]
                n470 = Delete From Array(array=w301, index (col)=0 ("disabled index (col)")) -> (deleted portion=w298:dbl[], array with subset deleted=w300:dbl[][])  [unwired: 2 in]
                n471 = Threshold 1D Array(2:w299, 3:w298) -> (0:w294:dbl)  [unwired: 1 in]
                n472 = To Long Integer(number=w294) -> (32bit integer=w293:i32)
                n473 = Index Array(array=w300, index (row)=w293, index (col)=1 ("disabled index (col)")) -> (element=w296:dbl)
                n474 = Index Array(array=w300, index (row)=w293, index (col)=2 ("disabled index (col)")) -> (element=w295:dbl)
                n475 = Index Array(array=w300, index (row)=w293, index (col)=0 ("disabled index (col)")) -> (element=w297:dbl)
              }
              frame True {
                w313 = 0 ("disabled index (col)")
                n476 = Decimal String To Number(string=w317, default (0L)=0.0) -> (number=w309:dbl[][])  [unwired: 1 in, 1 out]
                n477 = Index Array(array=w309, index (row)=w313, index (col)=1 ("disabled index (col)")) -> (element=w311:dbl)
                n478 = Index Array(array=w309, index (row)=w313, index (col)=2 ("disabled index (col)")) -> (element=w310:dbl)
                n479 = Index Array(array=w309, index (row)=w313, index (col)=w313) -> (element=w312:dbl)
              }
            }
            "new P 2" <- w269
            "new I 2" <- w268
            "new D 2" <- w267
            n480 = Bundle By Name(cluster=T8 {"Row"=0, "Column"=0} ("Selection Start"), "Row"=w273) -> (w264:T8)
            n481 = property on="PID auto tab 2" class="Tbl (strict)"("Selection Color"=u32 16860, "Selection Size"=T8 {"Row"=1, "Column"=4}, "Selection Start"=w264) -> ()  [unwired: 2 in, 2 out]
          }
        }
      }
      n482 = while {
        tunnel: [TRUE] -> w190
        stop <- w1175 stop-if-true
        # "Recipe control"
        n483 = event shown="[0] Timeout" {
          selector: _ -> [_ _]
          dyn-events: _ -> [_ _]
          timeout: 250 -> [_ _]
          event Timeout {
            n484 = event-data() -> ()  [unwired: 1 in, 3 out]
          }
          event "ResetActRamp": Value Change {
            n485 = event-data() -> ("OldVal"=w1211:bool, "NewVal"=w1210:bool)  [unwired: 1 in, 4 out]
            n486 = Not(x=w1211) -> (.not. x?=w1209:bool)
            n487 = local read "OperateButton"() -> (w1208:bool)
            n488 = local read "Adv.RampControl"() -> (w1207:bool)
            n489 = And(x=w1209, y=w1210) -> (x .and. y?=w1206:bool)
            n490 = Compound Arithmetic op=AND(w1208, w1207, w1206) -> (w1205:bool)
            n491 = case shown="True" w1205 {
              frame False {
              }
              frame True {
                n492 = stacked-sequence {
                  frame #0 {
                    n493 = local write "OperateButton"(FALSE) -> ()
                  }
                  frame #1 {
                    n494 = Wait Until Next ms Multiple(millisecond multiple=u32 510) -> ()  [unwired: 1 out]
                  }
                  frame #2 {
                    n495 = local write "OperateButton"(TRUE) -> ()
                  }
                }
              }
            }
          }
        }
        n496 = local read "Boolean"() -> (w1175:T2)
        n497 = case shown="True" "Adv.RampControl" {
          frame False {
          }
          frame True {
            w1194 = 1.1 ("y")
            n498 = local read "Target Ramp:"() -> (w1184:dbl)
            n499 = local read "Act. Ramp:"() -> (w1195:dbl)
            n500 = local read "heat_LastData"() -> (w1190:dbl[])
            n501 = Multiply(x=w1184, y=w1194) -> (x*y=w1193:dbl)
            n502 = Divide(x=w1184, y=w1194) -> (x/y=w1192:dbl)
            n503 = Index Array(array=w1190, index #1=0 ("index (row)"), index #2=1 ("index (row)")) -> (element #1=w1187:dbl, element #2=w1185:dbl)
            n504 = In Range and Coerce(upper limit=w1193, x=w1195, lower limit=w1192) -> (In Range?=w1177:bool)  [unwired: 1 out]
            n505 = local read "Text Ring 3"() -> (w1182:u16)
            n506 = Multiply(x=10.0 ("y"), y=w1184) -> (x*y=w1181:dbl)
            n507 = case shown="0, Default" w1182 {
              tunnel: w1181 -> [w1197 w1200 w1203]
              tunnel: [w1197 w1198 w1201] -> w1179
              frame 0, Default {
              }
              frame 1 {
                n508 = Divide(x=w1200, y=60.0) -> (x/y=w1198:dbl)
              }
              frame 2 {
                w1202 = 60.0 ("y")
                n509 = Divide(x=w1203, y=w1202) -> (x/y=w1204:dbl)
                n510 = Divide(x=w1204, y=w1202) -> (x/y=w1201:dbl)
              }
            }
            n511 = Add(x=w1185, y=w1179) -> (x+y=w1186:dbl)
            n512 = Subtract(x=w1185, y=w1179) -> (x-y=w1191:dbl)
            n513 = In Range and Coerce(upper limit=w1186, x=w1187, lower limit=w1191) -> (In Range?=w1180:bool)  [unwired: 1 out]
            n514 = Not(x=w1180) -> (.not. x?=w1178:bool)
            n515 = And(x=w1178, y=w1177) -> (x .and. y?=w1176:bool)
            n516 = case shown="False" w1176 {
              tunnel: w1176 -> [_ w1196]
              frame False {
              }
              frame True {
                n517 = property on="ResetActRamp" class="Bool (strict)"("Val(Sgnl)"=w1196) -> ()  [unwired: 2 in, 2 out]
              }
            }
          }
        }
      }
      n518 = while {
        tunnel: w178 -> [w1032]
        stop <- w1040 stop-if-true
        (unwired) u32 500 ("millisecond multiple")
        # "Graf loop"
        n519 = case shown="True" "Start 2" {
          tunnel: "Sampling time" -> [_ w1052]
          tunnel: w1032 -> [_ w1051]
          frame False {
          }
          frame True {
            n520 = local read "Ie Act.:"() -> (w1058:dbl)
            n521 = Select(t=0.0 ("y"), s=w1051, f=1000.0 ("y")) -> (s? t:f=w1048:dbl)
            n522 = Multiply(x=w1058, y=w1048) -> (x*y=w1060:dbl)
            n523 = local read "Uc Act.:"() -> (w1055:dbl)
            n524 = local read "Ue Act.:"() -> (w1056:dbl)
            n525 = local read "Ic Act.:"() -> (w1057:dbl)
            n526 = Bundle(cluster=T5 {"[0]"=0.0, "[1]"=0.0, "[2]"=0.0, "[3]"=0.0}, "[0]"=w1057, "[1]"=w1060, "[2]"=w1055, "[3]"=w1056) -> (→"main Graph 2":T5)
            n527 = Divide(x=w1052, y=1000.0) -> (x/y=w1053:dbl)
            n528 = property on="main Graph 2" class="WFChart (strict)"("XScale.Multiplier"=w1053) -> ()  [unwired: 2 in, 2 out]
          }
        }
        n529 = event shown="[6] \"Saveproject\": Value Change" {
          selector: _ -> [_ _ _ _ _ _ _ _ _]
          dyn-events: _ -> [_ _ _ _ _ _ _ _ _]
          timeout: 1 -> [_ _ _ _ _ _ _ _ _]
          tunnel: [_ w1081 _ w1092 _ _ _ _ _] -> w1040
          tunnel: T10 {"Name"="0", "Color"=16776960, "Style"=4, "Point Style"=3, "Name Visible"=FALSE, "Allow Drag"=TRUE, "Cursor Mode"=0, "Plot"=0, "Index"=0, "Position"={"X"=0.0, "Y"=0.0}, "X Scale"=0, "Y Scale"=0, "Watch Plots"=[], "Watch All Plots"=FALSE, "Plot Area"=0, "Label Offset"={"X"=1.0408340855860843e-17, "Y"=0.5847953216374269}} ("element") -> [_ _ _ _ _ _ _ w1143 _]
          event Timeout {
            # "Axies name:"
            n530 = event-data() -> ()  [unwired: 1 in, 3 out]
            n531 = property on="Temp. unit:" class="Ring (strict)"() -> ("RingText.Text"=w1077:string)  [unwired: 2 in, 2 out]
            n532 = Concatenate Strings("Temperature [" ("string"), w1077, "]" ("string")) -> (w1076:string)
            n533 = property on="Waveform Graph" class="WFGraph (strict)"("ActYScl"=0, "YScale.NameLbl.Text"=w1076) -> ()  [unwired: 2 in, 2 out]
          }
          event Panel Close {
            w1081 = TRUE
            n534 = event-data() -> ()  [unwired: 1 in, 4 out]
            n535 = while {
              tunnel: w1081 -> [w1083]
              stop <- w1084 stop-if-true
              n536 = local write "Boolean"(w1083) -> ()
              n537 = local read "stopped_loops"() -> (w1084:bool)
              n538 = Wait (ms)(milliseconds to wait=10) -> ()  [unwired: 1 out]
            }
          }
          event "Temp. unit:": Value Change {
            n539 = event-data() -> ()  [unwired: 1 in, 6 out]
            n540 = property on="Temp. unit:" class="Ring (strict)"() -> ("Strings []"=w1089:string[], "Value"=w1087:u16)  [unwired: 2 in, 2 out]
            n541 = Reverse 1D Array(array=w1089) -> (reversed array=w1088:string[])
            n542 = Index Array(array=w1088, index=w1087) -> (element=w1086:string)
            n543 = Concatenate Strings("Temperature [" ("string"), w1086, "]" ("string")) -> (w1085:string)
            n544 = property on="main Graph" class="WFChart (strict)"("YScale.NameLbl.Text"=w1085) -> ()  [unwired: 2 in, 2 out]
          }
          event "stop": Value Change {
            w1092 = TRUE
            n545 = event-data() -> ()  [unwired: 1 in, 6 out]
            n546 = while {
              tunnel: w1092 -> [w1093]
              stop <- w1095 stop-if-true
              n547 = local write "Boolean"(w1093) -> ()
              n548 = Wait (ms)(milliseconds to wait=10) -> ()  [unwired: 1 out]
              n549 = local read "stopped_loops"() -> (w1095:bool)
            }
          }
          event "Clear ALL": Value Change {
            n550 = event-data() -> ()  [unwired: 1 in, 6 out]
            n551 = property on="main Graph" class="WFChart (strict)"("History Data"=T11 []) -> ()  [unwired: 2 in, 2 out]
          }
          event "Save As Button": Value Change {
            w1108 = T16 2 items=["User Home"=0, "User Desktop"=1, "User Documents"=2, "User Application Data"=3, "User Preferences"=4, "User Temporary"=5, "Public Documents"=6, "Public Application Data"=7, "Public Preferences"=8, "Public Cache"=13, "System Core Libraries"=9, "System Installed Libraries"=10, "Application Files"=11, "Boot Volume Root"=12] ("system directory type")
            n552 = event-data() -> ()  [unwired: 1 in, 6 out]
            n553 = local read "Waveform Graph"() -> (w1101:waveform(dbl)[])
            n554 = Get Date/Time In Seconds() -> (seconds since 1Jan1904=w1106:timestamp)
            n555 = Format Date/Time String() -> ()  [unwired: 3 in, 1 out]
            n556 = Format Date/Time String(time format string (%c)="%H.%M.%S", seconds (now)=w1106) -> (date/time string=w1105:string)  [unwired: 1 in]
            n557 = call <vilib>:"Get System Directory.vi"("create directory if not found? (F)"=TRUE, "system directory type"=w1108) -> ("system directory"=w1107:path)  [unwired: 9 in]
            n558 = Concatenate Strings("TDS_" ("default name"), w1105, ".txt" ("default name")) -> (w1103:string)
            n559 = call "File Dialog"("start path"=w1107, "default name"=w1103) -> ("selected path"=w1097:path, "error out"=w1099:errorcluster)  [unwired: 10 in, 2 out]
            n560 = call-poly <vilib>:"Export Waveforms to Spreadsheet File.vi"("error in (no error)"=w1099, "waveforms"=w1101, "file path (dialog if empty)"=w1097) -> ("error out"=w1102:errorcluster)  [unwired: 7 in, 1 out]
            n561 = call <vilib>:"Clear Errors.vi"("error in (no error)"=w1102) -> ()  [unwired: 5 in, 2 out]
          }
          event "Saveproject": Value Change {
            n562 = event-data() -> ()  [unwired: 1 in, 6 out]
            n563 = local read "Regulation TYpe"() -> (w1118:bool)
            n564 = local read "Heating Mode:"() -> (w1115:bool)
            n565 = local read "Target Ue [V]:"() -> (w1117:dbl)
            n566 = local read "Target Ramp:"() -> (w1110:dbl)
            n567 = local read "Target Temp:"() -> (w1111:dbl)
            n568 = local read "Target Ic [A]:"() -> (w1116:dbl)
            n569 = local read "PID Output:"() -> (w1119:bool)
            n570 = local read "Temp. unit:"() -> (w1113:u16)
            n571 = local read "Ramp unit:"() -> (w1112:u16)
            n572 = Bundle By Name(cluster="TDS", "Target Temp:"=w1111, "Target Ramp:"=w1110, "Ramp unit:"=w1112, "Temp. unit:"=w1113, "Target Ue [V]:"=w1117, "Target Ic [A]:"=w1116, "Heating Mode:"=w1115, "PID Output:"=w1119, "Regulation Type"=w1118) -> (w1114:T1)
            n573 = call "File Dialog2"("default name"="TDS_ProcessConfig.json") -> ("selected path"=w1122:path, "cancelled"=w1121:bool)  [unwired: 11 in, 2 out]
            n574 = case shown="False" w1121 {
              tunnel: w1122 -> [w1124 _]
              tunnel: w1114 -> [w1136 _]
              frame False {
                w1125 = TRUE ("replace all? (F)")
                n575 = Flatten To JSON(anything=w1136) -> (JSON string=w1132:string, 11:w1133:errorcluster)  [unwired: 2 in]
                n576 = Search and Replace String(replace all?=w1125, input string=w1132, search string="},{", replace string="},\n{" ("search string"), error in=w1133) -> (result string=w1131:string, error out=w1127:errorcluster)  [unwired: 3 in, 2 out]
                n577 = Search and Replace String(replace all?=w1125, input string=w1131, search string=",\"", replace string=",\n    \"" ("search string"), error in=w1127) -> (result string=w1128:string, error out=w1126:errorcluster)  [unwired: 3 in, 2 out]
                n578 = Open/Create/Replace File(file path (use dialog)=w1124, error in=w1126, operation (0:open)=T12."replace or create with confirmation") -> (refnum out=w1141:refnum<file>, error out=w1140:errorcluster)  [unwired: 3 in, 1 out]
                n579 = Write to Text File(file (use dialog)=w1141, text=w1128, error in=w1140) -> (refnum out=w1139:refnum<file>, error out=w1138:errorcluster)  [unwired: 1 in, 1 out]
                n580 = Close File(refnum=w1139, error in=w1138) -> (error out=w1137:errorcluster)  [unwired: 1 out]
                n581 = call <vilib>:"Clear Errors.vi"("error in (no error)"=w1137) -> ()  [unwired: 5 in, 2 out]
              }
              frame True {
              }
            }
          }
          event "Loadproject": Value Change {
            n582 = event-data() -> ()  [unwired: 1 in, 6 out]
            n583 = call "File Dialog3"("default name"="TDS_ProcessConfig.json") -> ("selected path"=w1146:path, "exists"=w1144:bool, "cancelled"=w1145:bool)  [unwired: 11 in, 1 out]
            n584 = case shown="False" w1145 {
              tunnel: w1146 -> [w1149 _]
              tunnel: w1144 -> [w1150 _]
              tunnel: w1143 -> [w1148 _]
              frame False {
                n585 = case shown="True" w1150 {
                  tunnel: w1149 -> [_ w1162]
                  tunnel: w1148 -> [_ _]
                  frame False {
                  }
                  frame True {
                    n586 = Open/Create/Replace File(file path (use dialog)=w1162, operation (0:open)=T12."open") -> (refnum out=w1168:refnum<file>, error out=w1167:errorcluster)  [unwired: 4 in, 1 out]
                    n587 = Read from Text File(file (use dialog)=w1168, error in=w1167) -> (refnum out=w1163:refnum<file>, text=w1166:string, error out=w1164:errorcluster)  [unwired: 2 in, 1 out]
                    n588 = Unflatten From JSON(JSON string=w1166, type and defaults="TDS 2", error in (no error)=w1164) -> (value=w1160:T1, error out=w1165:errorcluster)  [unwired: 4 in]
                    n589 = Unbundle By Name(w1160) -> ("Target Temp:"=w1158:dbl, "Target Ramp:"=w1157:dbl, "Ramp unit:"=w1156:u16, "Temp. unit:"=w1159:u16, "Target Ue [V]:"=w1155:dbl, "Target Ic [A]:"=w1154:dbl, "Heating Mode:"=w1153:bool, "PID Output:"=w1152:bool, "Regulation Type"=w1151:bool)  [unwired: 2 out]
                    n590 = Close File(refnum=w1163, error in=w1165) -> (error out=w1169:errorcluster)  [unwired: 1 out]
                    n591 = local write "Temp. unit:"(w1159) -> ()
                    n592 = call <vilib>:"Clear Errors.vi"("error in (no error)"=w1169) -> ()  [unwired: 5 in, 2 out]
                    n593 = property on="Target Ramp:" class="DigNum (strict)"("Val(Sgnl)"=w1157) -> ()  [unwired: 2 in, 2 out]
                    n594 = property on="Target Ic [A]:" class="DigNum (strict)"("Val(Sgnl)"=w1154) -> ()  [unwired: 2 in, 2 out]
                    n595 = property on="PID Output:" class="Bool (strict)"("Val(Sgnl)"=w1152) -> ()  [unwired: 2 in, 2 out]
                    n596 = property on="Target Temp:" class="DigNum (strict)"("Val(Sgnl)"=w1158) -> ()  [unwired: 2 in, 2 out]
                    n597 = property on="Ramp unit:" class="Ring (strict)"("Val(Sgnl)"=w1156) -> ()  [unwired: 2 in, 2 out]
                    n598 = property on="Target Ue [V]:" class="DigNum (strict)"("Val(Sgnl)"=w1155) -> ()  [unwired: 2 in, 2 out]
                    n599 = property on="Heating Mode:" class="Bool (strict)"("Val(Sgnl)"=w1153) -> ()  [unwired: 2 in, 2 out]
                    n600 = property on="Regulation TYpe" class="Bool (strict)"("Val(Sgnl)"=w1151) -> ()  [unwired: 2 in, 2 out]
                  }
                }
              }
              frame True {
              }
            }
          }
          event "Clear ALL 2": Value Change {
            n601 = event-data() -> ()  [unwired: 1 in, 6 out]
            n602 = property on="main Graph 2" class="WFChart (strict)"("History Data"=T13 []) -> ()  [unwired: 2 in, 2 out]
          }
        }
        n603 = Wait Until Next ms Multiple(millisecond multiple="Sampling time") -> ()  [unwired: 1 out]
        n604 = case shown="True" "Start 1" {
          frame False {
          }
          frame True {
            (unwired) 0.5 ("y")
            n605 = Get Date/Time In Seconds() -> (seconds since 1Jan1904=w1066:timestamp)
            n606 = local read "Sampling time"() -> (w1064:dbl)
            n607 = property on="main Graph" class="WFChart (strict)"() -> ("History Data"=w1069:T11)  [unwired: 2 in, 2 out]
            n608 = for {
              tunnel: w1069 -> [w1075] mode=indexing
              tunnel: [w1074] -> w1068 mode=indexing
              n609 = Cluster To Array(cluster=w1075) -> (array=w1074:dbl[])
            }
            n610 = Divide(x=w1064, y=1000.0) -> (x/y=w1063:dbl)
            n611 = Transpose 2D Array(2D array=w1068) -> (transposed array=w1067:dbl[][])
            n612 = for {
              tunnel: w1066 -> [w1073]
              tunnel: w1063 -> [w1072]
              tunnel: w1067 -> [w1071] mode=indexing
              tunnel: [w1070] -> w1065 mode=indexing
              n613 = Bundle By Name("Y"=w1071, "dt"=w1072, "t0"=w1073) -> (w1070:waveform(dbl))  [unwired: 1 out]
            }
            "Waveform Graph" <- w1065
          }
        }
        n614 = local read "heat_LastData"() -> (w1034:dbl[])
        n615 = case shown="True" w1032 {
          tunnel: w1034 -> [w1042 w1047]
          tunnel: [w1042 w1043] -> w1033
          frame False {
          }
          frame True {
            n616 = local read "Act. Setpoint: 2"() -> (w1044:dbl)
            n617 = local read "Act. Temp:"() -> (w1045:dbl)
            n618 = Build Array(w1045, w1044) -> (w1046:dbl[])
            n619 = Build Array (concatenate)(w1047, w1046) -> (w1043:dbl[])
          }
        }
        n620 = Array To Cluster(array=w1033) -> (cluster=→"main Graph":T4)
      }
      n621 = Compound Arithmetic op=AND(w190, w182) -> (w199:bool)
      n622 = local write "stopped_loops"(w199) -> ()
      n623 = call-dynamic "Write Single Holding Register.vi"("error in (no error)"=w193, "holding register value"=u16 1, "address"=u16 71, "Modbus master in"=w194) -> ("error out"=w191:errorcluster, "Modbus master out"=w192:refnum<class "Modbus Master.lvclass">)  [unwired: 6 in]
      n624 = call-dynamic "Close.vi"("error in (no error)"=w191, "Modbus master in"=w192) -> ("error out"=w183:errorcluster)  [unwired: 9 in]
      n625 = call <vilib>:"Clear Errors.vi"("error in (no error)"=w183) -> ()  [unwired: 5 in, 2 out]
    }
    frame #2 {
      w1223 = "DualDC"  # Key 3
      w1224 = "Others" ("section")
      w1231 = "Shutter Control"  # Key 3
      w1233 = "%s" ("format string")
      w1238 = "HEAT3 PID manual tab"  # Key 3
      w1239 = "HEAT3 PID tab 2"  # Key 2
      w1250 = "HEAT3 Sampling time"  # Key 1
      w1258 = "HEAT3 PID manual tab"  # Key 3
      w1264 = "HEAT3 PID tab 1"  # Key 2
      w1254 = "Section 2"
      w1266 = "HEAT3 Path"  # Key 1
      w1247 = "Section 1"
      n626 = local read "PID manual setting"() -> (w1256:string[][])
      n627 = local read "Sampling time"() -> (w1248:dbl)
      n628 = local read "PID auto tab"() -> (w1261:string[][])
      n629 = local read "PID manual setting 2"() -> (w1234:string[][])
      n630 = local read "PID auto tab 2"() -> (w1235:string[][])
      n631 = local read "address"() -> (w1265:string)
      n632 = call <vilib>:"Application Directory.vi"() -> ("Application Directory"=w1252:path)
      n633 = Build Path(base path=w1252, name or relative path="TDS Configuration File.ini") -> (appended path=w1251:path)
      n634 = Number To Fractional String(number=w1248) -> (F-format string=w1249:string)  [unwired: 3 in]
      n635 = Array To Spreadsheet String(array=w1261, 3:"%s" ("format string")) -> (spreadsheet string=w1263:string)  [unwired: 1 in]
      n636 = Array To Spreadsheet String(array=w1256, 3:"%s" ("format string")) -> (spreadsheet string=w1255:string)  [unwired: 1 in]
      n637 = Delete(path (use dialog)=w1251) -> (deleted path=w1269:path)  [unwired: 4 in, 2 out]
      n638 = call <vilib>:"Open Config Data.vi"("configuration file path"=w1269) -> ("error out"=w1267:errorcluster, "refnum"=w1268:T15)  [unwired: 2 in, 7 out]
      n639 = call-poly <vilib>:"Write Key.vi"("section"=w1247, "error in (no error)"=w1267, "value"=w1265, "key"=w1266, "refnum"=w1268) -> ("error out"=w1245:errorcluster, "refnum out"=w1246:T15)  [unwired: 1 in, 4 out]
      n640 = call-poly <vilib>:"Write Key.vi"("section"=w1247, "error in (no error)"=w1245, "value"=w1249, "key"=w1250, "refnum"=w1246) -> ("error out"=w1243:errorcluster, "refnum out"=w1244:T15)  [unwired: 1 in, 4 out]
      n641 = call-poly <vilib>:"Write Key.vi"("section"=w1254, "error in (no error)"=w1243, "value"=w1263, "key"=w1264, "refnum"=w1244) -> ("error out"=w1259:errorcluster, "refnum out"=w1260:T15)  [unwired: 1 in, 4 out]
      n642 = call-poly <vilib>:"Write Key.vi"("section"=w1254, "error in (no error)"=w1259, "value"=w1255, "key"=w1258, "refnum"=w1260) -> ("error out"=w1240:errorcluster, "refnum out"=w1241:T15)  [unwired: 1 in, 4 out]
      n643 = Array To Spreadsheet String(array=w1235, 3:w1233) -> (spreadsheet string=w1237:string)  [unwired: 1 in]
      n644 = Array To Spreadsheet String(array=w1234, 3:w1233) -> (spreadsheet string=w1236:string)  [unwired: 1 in]
      n645 = local read "ShutterControl"() -> (w1228:bool)
      n646 = Select(t="True" ("format string"), s=w1228, f="False" ("format string")) -> (s? t:f=w1225:string)
      n647 = local read "DualDC"() -> (w1215:bool)
      n648 = case shown="True" w1215 {
        tunnel: "Section 3" -> [_ w1280]
        tunnel: w1241 -> [w1271 w1279]
        tunnel: w1240 -> [w1270 w1278]
        tunnel: [w1271 w1277] -> w1230
        tunnel: [w1270 w1276] -> w1229
        tunnel: w1239 -> [_ w1275]
        tunnel: w1238 -> [_ w1274]
        tunnel: w1237 -> [_ w1273]
        tunnel: w1236 -> [_ w1272]
        frame False {
        }
        frame True {
          n649 = call-poly <vilib>:"Write Key.vi"("section"=w1280, "error in (no error)"=w1278, "value"=w1273, "key"=w1275, "refnum"=w1279) -> ("error out"=w1281:errorcluster, "refnum out"=w1282:T15)  [unwired: 1 in, 4 out]
          n650 = call-poly <vilib>:"Write Key.vi"("section"=w1280, "error in (no error)"=w1281, "value"=w1272, "key"=w1274, "refnum"=w1282) -> ("error out"=w1276:errorcluster, "refnum out"=w1277:T15)  [unwired: 1 in, 4 out]
        }
      }
      n651 = call-poly <vilib>:"Write Key.vi"("section"=w1224, "error in (no error)"=w1229, "value"=w1225, "key"=w1231, "refnum"=w1230) -> ("error out"=w1219:errorcluster, "refnum out"=w1218:T15)  [unwired: 1 in, 4 out]
      n652 = Select(t="True" ("format string"), s=w1215, f="False" ("format string")) -> (s? t:f=w1220:string)
      n653 = call-poly <vilib>:"Write Key.vi"("section"=w1224, "error in (no error)"=w1219, "value"=w1220, "key"=w1223, "refnum"=w1218) -> ("error out"=w1216:errorcluster, "refnum out"=w1217:T15)  [unwired: 1 in, 4 out]
      n654 = call <vilib>:"Close Config Data.vi"("error in (no error)"=w1216, "refnum"=w1217) -> ("error out"=w1242:errorcluster)  [unwired: 1 in, 8 out]
      n655 = call <vilib>:"Clear Errors.vi"("error in (no error)"=w1242) -> ()  [unwired: 5 in, 2 out]
    }
  }
  "Connected:" <- w14
  "Comunication error:" <- w14
